vi "ME_acquire_12_DeltaForce_Daq.vi"() -> ()   [LabVIEW 2015]
doc: "Use this template to build a producer/consumer design pattern. Use this template when you need to execute a process, such as data analysis, when a data source, such as a triggered acquisition, produces data at an uneven rate and you need to execute the process when the data becomes available."
uses:
  Mode.ctl
  oxford_driver/Oxford Drivers/BUSGEN.LLB/OxfordAddress.ctl
  <vilib>/Analysis/baseanly.llb/Mean (DBL).vi
  <vilib>/DAQmx/read.llb/DAQmx Read (Analog 1D DBL 1Chan NSamp).vi
  <vilib>/Utility/file.llb/Write Delimited Spreadsheet (DBL).vi
  <vilib>/DAQmx/create/channels.llb/DAQmx Create Channel (AI-Voltage-Basic).vi
  <vilib>/DAQmx/configure/timing.llb/DAQmx Timing (Sample Clock).vi
  <vilib>/DAQmx/miscellaneous.llb/DAQmx Fill In Error Info.vi
  <vilib>/express/express arith-compare/Formula/XNode/ExpressFormulaBlockNode.xnode
  <vilib>/Analysis/NI_AALBase.lvlib
panel:
  out "mean":dbl format="%0.6f"
  out "remaining elements":T1(array[cluster])
  in  "Number of Samples":i32=100
  in  "Sample Rate":dbl=1000.0
  in  "Terminal Configuration":i32(ring)=-1 items=["default"=-1, "RSE"=10083, "NRSE"=10078, "Differential"=10106, "Pseudodifferential"=12529]
  in  "Max Voltage":dbl=5.0
  in  "Min Voltage":dbl=-5.0
  in  "Physical Channel":tag="Dev1/ai0"
  out "MagnetoRes (Ohm)":dbl
  in  "Averaged dt":dbl[][](array[numeric])
  in  "Averaged P(B)":dbl[][](array[numeric])
  out "LockInR":dbl
  out "deltaUaux":dbl
  out "Actual Voltage (V)":dbl caption="Actual AuxV" step=0.1
  in  "Stop":bool
  out "SaveSweep":bool=TRUE
  out "Measurement File_dn":path
  out "Measurement File_up":path
  out "Measurement File_average":path
  out "Actual Polarization":dbl
  in  "Reset IB?":bool
  in  "First?":bool
  in  "Save Period":dbl=1.0
  out "Averaged I(B)":dbl[][](array[numeric])
  out "P(uC/mm^2)":dbl[](array[numeric])
  in  "Sweep":bool
  out "Offset array":dbl[](array[numeric])
  in  "stop 2":bool
  in  "dB":dbl=0.005
  in  "Dwell Time (ms)":u32=1
  out "appended array":dbl[][](array[numeric])
  out "Actual B Field (T)":dbl
  out "Actual Temperature (K)":dbl
  out "Actual Current (pA)":dbl
  in  "Tab Control":T2(tab)
  in  "Max temperature (K)":dbl=20.0
  in  "Min Temperature (K)":dbl=4.5
  out "P(T)":cluster{"yi":dbl[], dbl[]}(graph)
  out "I(T)":cluster{dbl[], dbl[]}(graph)
  in  "Set temperature (K)":dbl=4.5
  in  "Temp Ramping Rate (K/min)":dbl=10.0
  in  "Heater Range":enum16{"Off", "Low", "Medium", "High"}(ring)
  in  "Heater On/Off":bool
  out "Setpoint Temperature (K)":dbl
  in  "FileName":string
  out "Step Temp":bool
  out "j":i32
  out "i":i32
  in  "Max Countl":i32
  in  "Record ALL":bool
  in  "Sweep Rate Array":dbl[](array[numeric])=[2.0, 1.0, 0.5, 0.1, 0.05, 9.0, 10.0, 11.0, 12.0]
  out "I(B) 3":cluster{dbl[], dbl[]}[](graph)
  in  "Go to Set":bool
  in  "Set Field (T)":dbl
  in  "Field To Zero":bool
  in  "Sweep Rate (T/min)":dbl=2.0 format="%.6f"
  in  "Min Field (T)":dbl
  in  "Max Field (T)":dbl=0.15
  out "Up/Down":bool
  out "I(B) /Averaged/":cluster{"B array":dbl[], dbl[]}[](graph)
  in  "Temperature Array":dbl[](array[numeric])=[4.5, 5.0, 6.0, 7.0, 8.0, 9.0, 10.0, 11.0, 12.0]
  out "New":bool=TRUE
  out "Step Rate":bool
  out "Finished":bool=TRUE
  in  "Directory":string
  out "Wait (s)":dbl
  in  "secs to wait":dbl=180.0
  in  "Max count array":i32[](array[numeric])=[2, 1, 0, 0, 0, 9, 10, 11, 12]
  out "Target Field":dbl
  out "P(B) /Averaged/":cluster{"B array":dbl[], dbl[]}[](graph)
  out "P(B)":cluster{"yi":dbl[], dbl[]}(graph)
  in  "Measure Noise":bool
  in  "Cycles":i32
  in  "maximum value":dbl=10.0 format="%0.2f"
  in  "minimum value":dbl=-10.0 format="%0.2f"
  in  "physical channels":tag="Dev1/ai1"
  out "PSD (pA/Hz^1/2) Peaks Removed":cluster{"f0":dbl, "df":dbl, "magnitude":dbl[]}(graph)
  out "PSD (pA/Hz^1/2)":cluster{"f0":dbl, "df":dbl, "magnitude":dbl[]}(graph)
  out "Current (pA) Filtered":waveform(dbl)(graph)
  out "Current (pA)":dbl[](graph)
  in  "Samples per channel":i32=1000
  in  "Rate":dbl=1000.0 format="%0.2f"
  in  "Cut-Off Frequency":dbl=100.0 caption="Lower Cut-Off"
  in  "Filter On":bool
  in  "Lock_in_Amplifier":refnum<visa-resource-name>="GPIB0::5::INSTR"
  out "Dc offset":dbl
  in  "Calibrate":bool
  in  "IV converter":refnum<visa-resource-name>="GPIB0::20::INSTR"
  in  "Magnetic Field":refnum<visa-resource-name>="GPIB0::21::INSTR"
  out "Time Lag":dbl=0.0500025749206543
  in  "Lake Shore":refnum<visa-resource-name>="GPIB0::11::INSTR"
  in  "Temp Refresh (s)":dbl=0.1
  in  "Sampling rate (Hz)":dbl=10.0
  in  "Gain (V/A)":dbl=1000000000.0
  in  "Sample area (mm^2)":dbl=3.9
  out "B_V":cluster{dbl[], "Best Linear Fit":dbl[]}[](graph)=[{[-0.00854253601, 0.00626134724, 0.0219834428, 0.0379117736, 0.0535871506, 0.0694316728, 0.0851615152, 0.100816481, 0.116478038, 0.132148461, 0.147876163, 0.16341701, 0.178976744, 0.194563632, 0.210251739, 0.225738944, 0.241298253, 0.256806034, 0.272344374, 0.287933477, 0.303494709, 0.318997125, 0.334591297, 0.350146681, 0.365618053, 0.380940961, 0.39666457, 0.412213675, 0.427724671, 0.443221444, 0.458760641, 0.474360042, 0.489915118, 0.505330598, 0.520967119, 0.536347531, 0.551813711, 0.567441155, 0.582995861, 0.598507522, 0.614041988, 0.629563151, 0.645106262, 0.660611914, 0.676136149, 0.691553948, 0.7071244, 0.72262999, 0.738171137, 0.753700392, 0.76919513, 0.784778028, 0.800215944, 0.8156961, 0.831325434, 0.846852183, 0.862326812, 0.877819169, 0.893312568, 0.90888536, 0.924354789], "Best Linear Fit"=[0.0, 0.005, 0.01, 0.015, 0.02, 0.025, 0.03, 0.035, 0.04, 0.045, 0.05, 0.055, 0.06, 0.065, 0.07, 0.075, 0.08, 0.085, 0.09, 0.095, 0.1, 0.105, 0.11, 0.115, 0.12, 0.125, 0.13, 0.135, 0.14, 0.145, 0.15, 0.155, 0.16, 0.165, 0.17, 0.175, 0.18, 0.185, 0.19, 0.195, 0.2, 0.205, 0.21, 0.215, 0.22, 0.225, 0.23, 0.235, 0.24, 0.245, 0.25, 0.255, 0.26, 0.265, 0.27, 0.275, 0.28, 0.285, 0.29, 0.295, 0.3]}, {[-0.00854253601, 0.00626134724, 0.0219834428, 0.0379117736, 0.0535871506, 0.0694316728, 0.0851615152, 0.100816481, 0.116478038, 0.132148461, 0.147876163, 0.16341701, 0.178976744, 0.194563632, 0.210251739, 0.225738944, 0.241298253, 0.256806034, 0.272344374, 0.287933477, 0.303494709, 0.318997125, 0.334591297, 0.350146681, 0.365618053, 0.380940961, 0.39666457, 0.412213675, 0.427724671, 0.443221444, 0.458760641, 0.474360042, 0.489915118, 0.505330598, 0.520967119, 0.536347531, 0.551813711, 0.567441155, 0.582995861, 0.598507522, 0.614041988, 0.629563151, 0.645106262, 0.660611914, 0.676136149, 0.691553948, 0.7071244, 0.72262999, 0.738171137, 0.753700392, 0.76919513, 0.784778028, 0.800215944, 0.8156961, 0.831325434, 0.846852183, 0.862326812, 0.877819169, 0.893312568, 0.90888536, 0.924354789], "Best Linear Fit"=[-0.00022554388023060128, 0.004536267537808887, 0.009593430775915074, 0.014716931562355689, 0.01975906732634002, 0.024855610270593523, 0.029915265354287977, 0.03495083565949541, 0.03998852608757118, 0.045029068349812316, 0.05008803495326229, 0.055086897848955874, 0.060091835929837946, 0.06510550835596321, 0.07015173884687344, 0.07513334727738563, 0.08013814865293042, 0.08512637555172443, 0.0901244320467579, 0.09513881694893507, 0.10014423687592358, 0.10513073807087174, 0.11014675346564809, 0.1151502923271957, 0.12012680792099008, 0.1250555686413888, 0.1301132186920259, 0.13511473785283767, 0.14010399888730068, 0.14508868495702945, 0.1500870171143548, 0.15510471446726903, 0.16010815425765457, 0.16506669165212906, 0.17009632901003072, 0.1750435864450521, 0.18001843198211442, 0.1850451496356715, 0.19004847041199868, 0.1950379453501071, 0.20003475573578386, 0.20502728708357412, 0.21002687821664084, 0.21501442030211, 0.220007939788244, 0.2249672231113706, 0.22997560874002893, 0.23496313088260184, 0.23996209027618054, 0.24495722449359253, 0.24994125598600042, 0.2549536449902534, 0.25991939913989753, 0.2648987401917687, 0.26992606578200207, 0.2749203939204135, 0.2798979571595809, 0.2848812227804405, 0.2898648235706211, 0.2948739618827834, 0.2998498524919418]}]
  out "V_I":cluster{dbl[], "Best Linear Fit":dbl[]}[](graph)=[{[0.0, 0.035, 0.069, 0.104, 0.138, 0.173, 0.208, 0.242, 0.277, 0.311, 0.346, 0.38, 0.415, 0.45, 0.484, 0.519, 0.553, 0.588, 0.623, 0.657, 0.692, 0.726, 0.761, 0.796, 0.83, 0.865, 0.899, 0.934, 0.969, 1.003, 1.038, 1.072, 1.107, 1.141, 1.176, 1.211, 1.245, 1.28, 1.314, 1.349, 1.384, 1.418, 1.453, 1.487, 1.522, 1.557, 1.591, 1.626, 1.66, 1.695, 1.73, 1.764, 1.799, 1.833, 1.868, 1.902, 1.937, 1.972, 2.006, 2.041, 2.075], "Best Linear Fit"=[-0.00854253601, 0.00626134724, 0.0219834428, 0.0379117736, 0.0535871506, 0.0694316728, 0.0851615152, 0.100816481, 0.116478038, 0.132148461, 0.147876163, 0.16341701, 0.178976744, 0.194563632, 0.210251739, 0.225738944, 0.241298253, 0.256806034, 0.272344374, 0.287933477, 0.303494709, 0.318997125, 0.334591297, 0.350146681, 0.365618053, 0.380940961, 0.39666457, 0.412213675, 0.427724671, 0.443221444, 0.458760641, 0.474360042, 0.489915118, 0.505330598, 0.520967119, 0.536347531, 0.551813711, 0.567441155, 0.582995861, 0.598507522, 0.614041988, 0.629563151, 0.645106262, 0.660611914, 0.676136149, 0.691553948, 0.7071244, 0.72262999, 0.738171137, 0.753700392, 0.76919513, 0.784778028, 0.800215944, 0.8156961, 0.831325434, 0.846852183, 0.862326812, 0.877819169, 0.893312568, 0.90888536, 0.924354789]}, {[0.0, 0.035, 0.069, 0.104, 0.138, 0.173, 0.208, 0.242, 0.277, 0.311, 0.346, 0.38, 0.415, 0.45, 0.484, 0.519, 0.553, 0.588, 0.623, 0.657, 0.692, 0.726, 0.761, 0.796, 0.83, 0.865, 0.899, 0.934, 0.969, 1.003, 1.038, 1.072, 1.107, 1.141, 1.176, 1.211, 1.245, 1.28, 1.314, 1.349, 1.384, 1.418, 1.453, 1.487, 1.522, 1.557, 1.591, 1.626, 1.66, 1.695, 1.73, 1.764, 1.799, 1.833, 1.868, 1.902, 1.937, 1.972, 2.006, 2.041, 2.075], "Best Linear Fit"=[-0.007846580254753975, 0.007882153481927697, 0.02316149482613275, 0.03889022856281441, 0.054169569907019474, 0.06989830364370113, 0.08562703738038281, 0.10090637872458785, 0.11663511246126955, 0.1319144538054746, 0.14764318754215625, 0.1629225288863613, 0.17865126262304296, 0.19437999635972467, 0.2096593377039297, 0.22538807144061138, 0.24066741278481643, 0.25639614652149806, 0.27212488025817977, 0.2874042216023848, 0.3031329553390665, 0.31841229668327153, 0.3341410304199532, 0.3498697641566349, 0.3651491055008399, 0.3808778392375216, 0.39615718058172666, 0.4118859143184083, 0.42761464805509, 0.442893989399295, 0.45862272313597674, 0.4739020644801818, 0.48963079821686345, 0.5049101395610684, 0.5206388732977502, 0.5363676070344319, 0.5516469483786369, 0.5673756821153185, 0.5826550234595236, 0.5983837571962053, 0.6141124909328869, 0.629391832277092, 0.6451205660137737, 0.6603999073579787, 0.6761286410946604, 0.691857374831342, 0.7071367161755471, 0.7228654499122288, 0.7381447912564338, 0.7538735249931156, 0.7696022587297972, 0.7848816000740022, 0.8006103338106839, 0.815889675154889, 0.8316184088915707, 0.8468977502357756, 0.8626264839724573, 0.878355217709139, 0.893634559053344, 0.9093632927900257, 0.9246426341342309]}]
  out "B0 (T)":dbl=0.0025222449819540214
  out "B/V (T/V)":dbl=0.321659617116981
  out "I0 (A)":dbl=-0.007846580254753975
  out "V/I (Ohm)":dbl=0.44939239247661916
  in  "Offset?":bool
  in  "Magnet":bool
  in  "Ramp":bool=TRUE
  out "MagnetoResistance (Ohm)":cluster{dbl[], dbl[]}(graph)
  in  "Temp/Magnetic Field":bool
  out "index":i8
  out "Read?":bool
  out "Magnetic Field (T)":dbl[](array[numeric])
  out "Reset":bool
  out "Measured Current (pA)":dbl[](array[numeric])
  out "Elapsed Time (s)":dbl[](array[numeric])
  out "Start time":timestamp
  in  "Enum":T3=enum."Process"
  out "B array":dbl[](array[numeric])
  in  "dB (T)":dbl=0.0025
  in  "Counter":i8
  out "L magnet (H)":dbl
  out "R magnet (mOhm)":dbl
  out "Actual Current (R0)":dbl
  out "Actual Field (T)":dbl
  out "Temperature array":dbl[](array[numeric])
  in  "New Measurement File":bool
  out "Measurement File":path
  out "refnum out":refnum<file>
  in  "Measuring":bool
  in  "Measure /Pause":bool
  in  "stop":bool
  # "DeltaForce"
  # "Discrete"
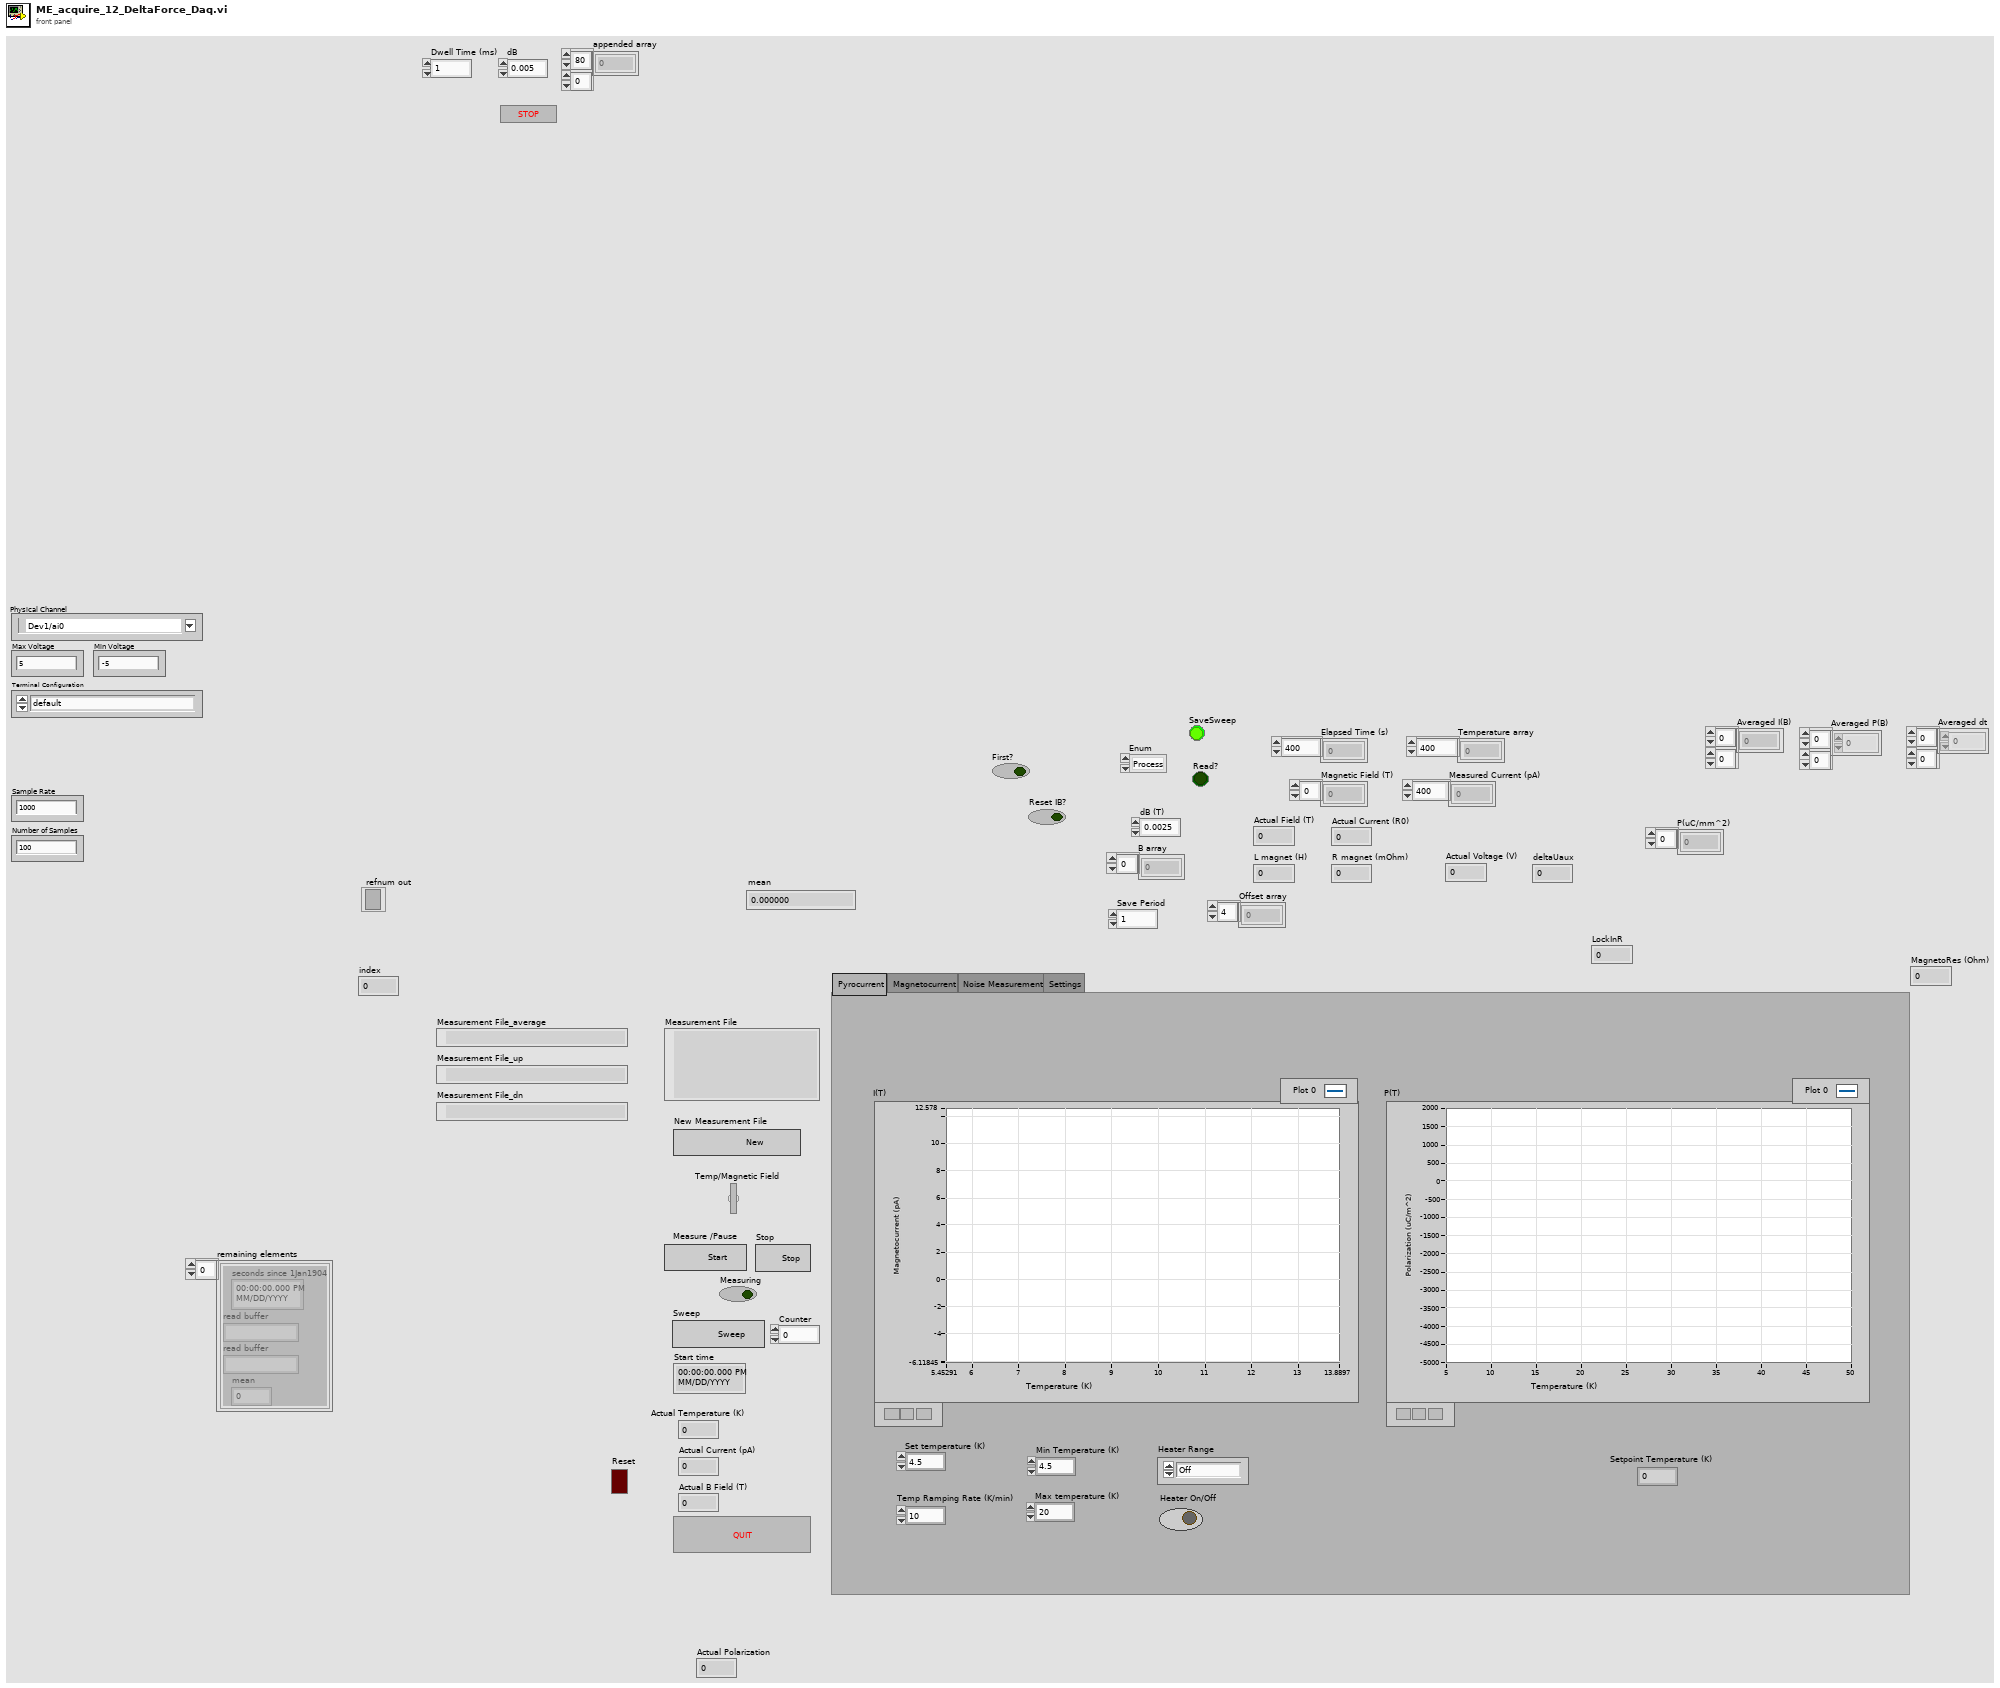
[diagram p1: front panel]
types:
  T1 = cluster{"seconds since 1Jan1904":timestamp, "read buffer":string, "read buffer":string, "mean":dbl}[]
  T2 = enum32{"Pyrocurrent", "Magnetocurrent", "Noise Measurement", "Settings"}
  T3 = typedef "Mode.ctl" = enum16{"Offset", "Process", "Sweep", "StepField", "Plot", "Save", "New", "Return", ""}
  T4 = cluster{"seconds since 1Jan1904":timestamp, "read buffer":string, "read buffer":string, "mean":dbl}
  T5 = enum16{"open", "replace", "create", "open or create", "replace or create", "replace or create with confirmation"}
  T6 = typedef "OxfordAddress.ctl" = cluster{"Com Port":i32, "ISOBUS Address":i32, "GPIB Address":i16, "Communication":enum16{"RS232", "ISOBUS", "GPIB", "Gateway"}}
  T7 = cluster{"B array":dbl[], "Averaged P(B) Out":dbl[]}
  T8 = cluster{"B array":dbl[], "Averaged I(B) out":dbl[]}
  T9 = cluster{"B array":dbl[], "Averaged P(B) Out":dbl[]}[]
  T10 = cluster{"B array":dbl[], "Averaged I(B) out":dbl[]}[]
  T11 = cluster{"I array out (A)":dbl[], "V array out (V)":dbl[]}
  T12 = cluster{"I array out (A)":dbl[], "Best Linear Fit":dbl[]}
  T13 = cluster{"V array out (V)":dbl[], "B array Out":dbl[]}
  T14 = cluster{"V array out (V)":dbl[], "Best Linear Fit 2":dbl[]}
  T15 = cluster{"I array out (A)":dbl[], "Best Linear Fit":dbl[]}[]
  T16 = cluster{"V array out (V)":dbl[], "Best Linear Fit 2":dbl[]}[]
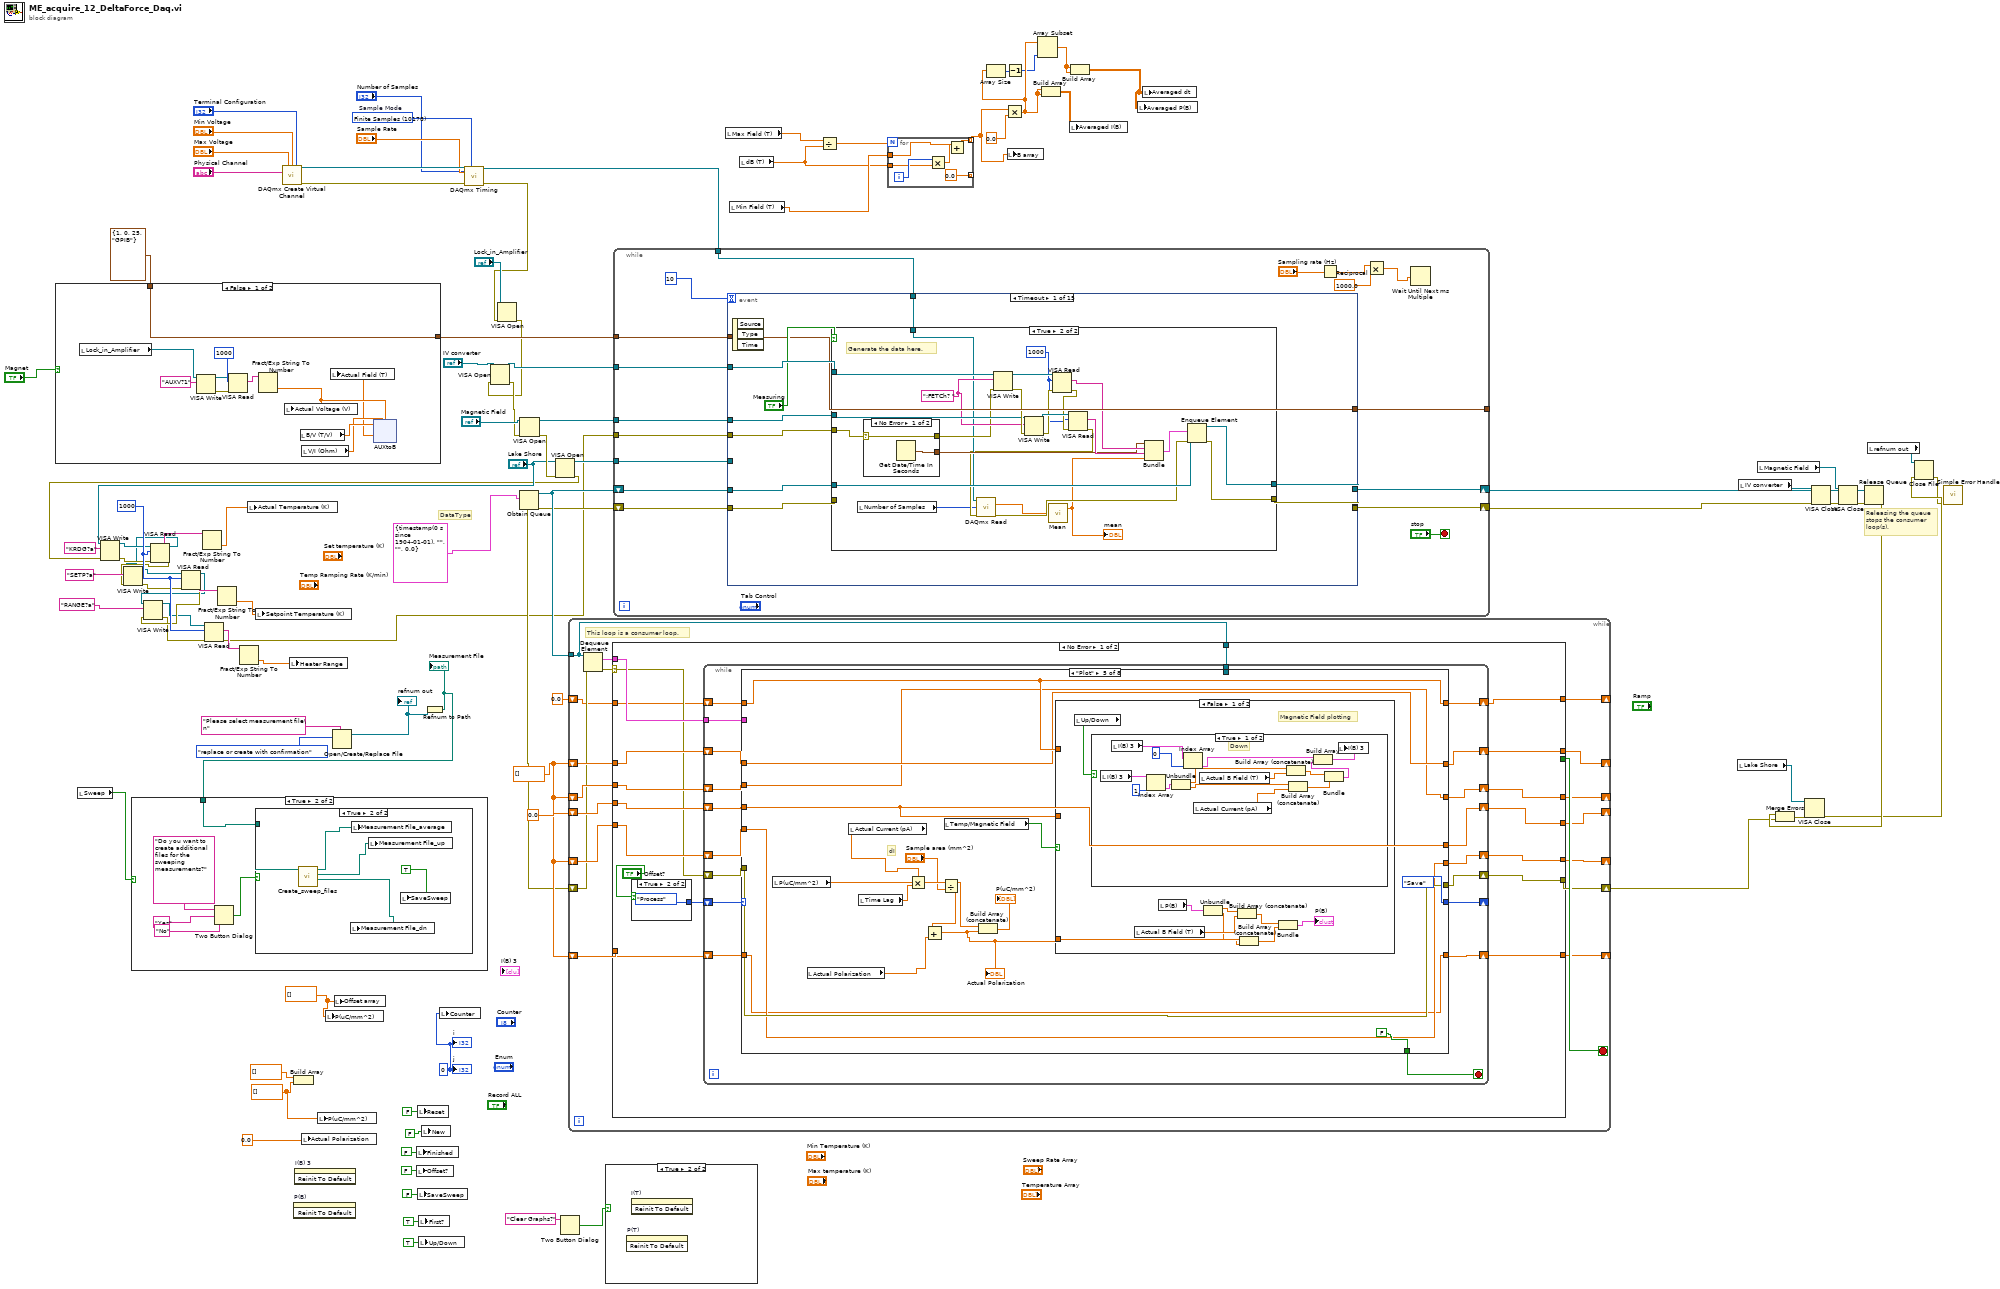
[diagram p0: block diagram]
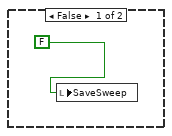
[diagram p4: hidden frame]
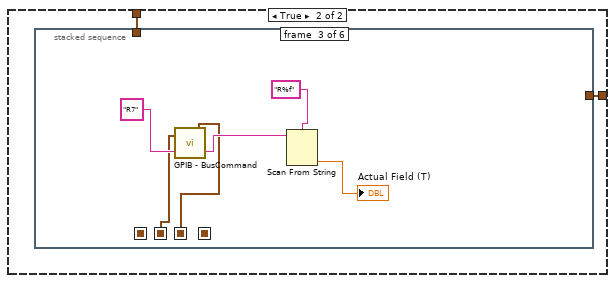
[diagram p5: hidden frame]
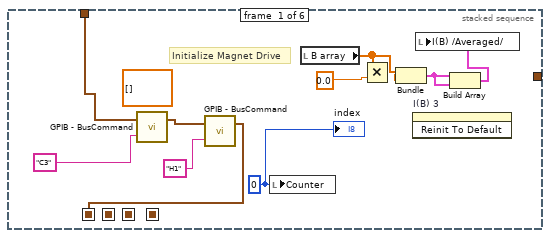
[diagram p6: hidden frame]
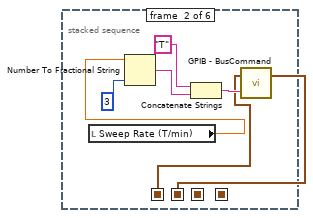
[diagram p7: hidden frame]
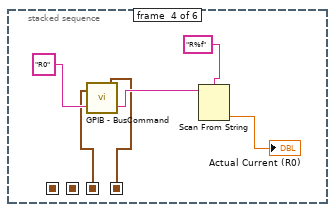
[diagram p8: hidden frame]
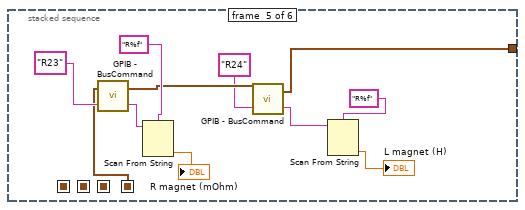
[diagram p9: hidden frame]
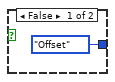
[diagram p11: hidden frame]
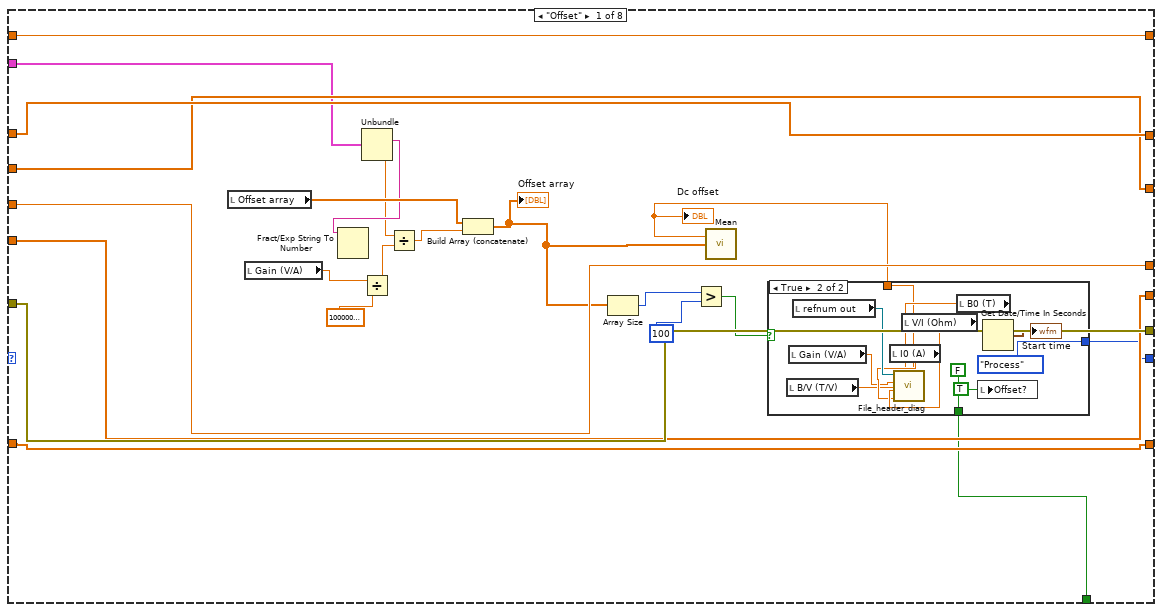
[diagram p12: hidden frame]
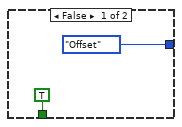
[diagram p13: hidden frame]
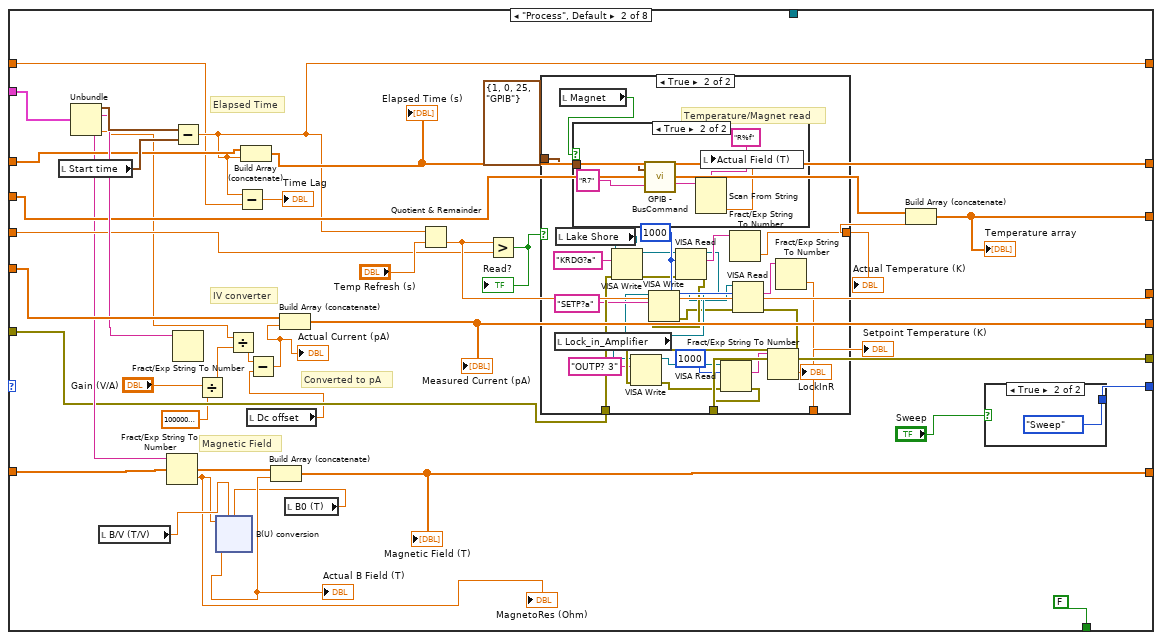
[diagram p14: hidden frame]
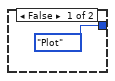
[diagram p15: hidden frame]
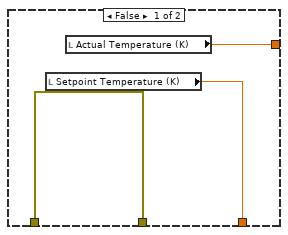
[diagram p16: hidden frame]
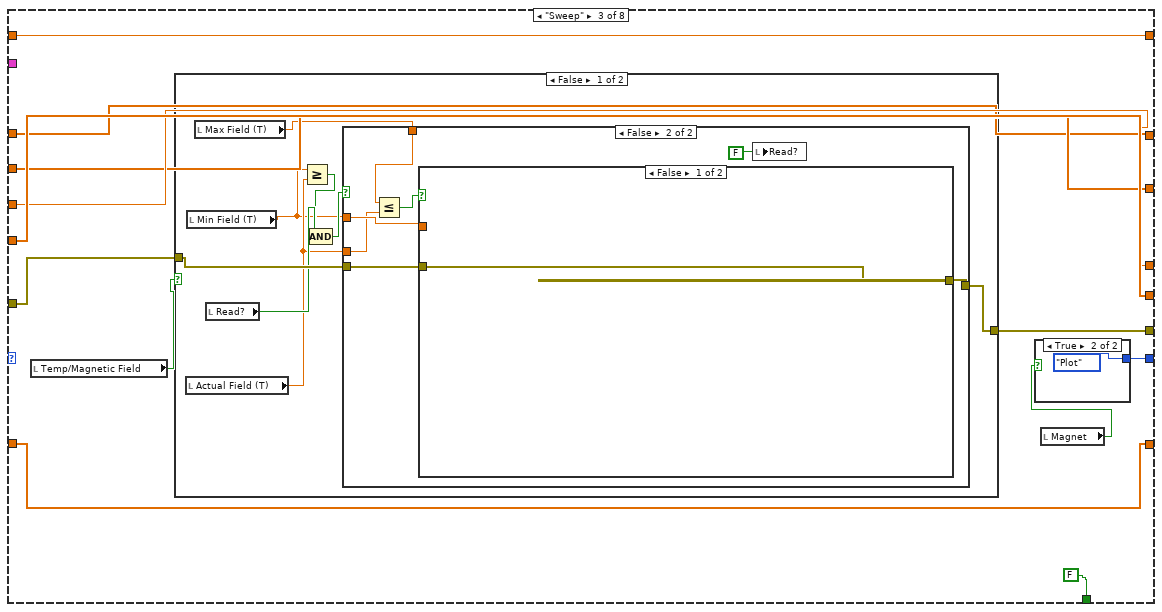
[diagram p18: hidden frame]
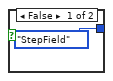
[diagram p19: hidden frame]
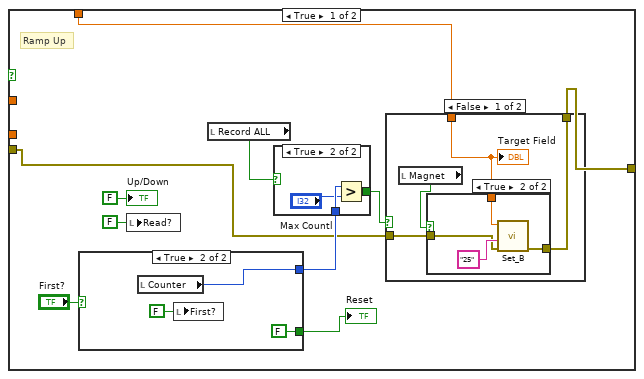
[diagram p20: hidden frame]
diagram:
  w9 = 10178 items=["Finite Samples"=10178, "Continuous Samples"=10123, "Hardware Timed Single Point"=12522]  # Sample Mode
  w39 = u32 1000 ("byte count")
  w50 = 0 ("j")
  w47 = dbl[] []
  w65 = dbl[] []
  w71 = dbl[] []
  # "DataType"
  # "Releasing the queue stops the consumer loop(s)."
  n1 = case shown="False" "Magnet" {
    tunnel: T6 {"Com Port"=1, "ISOBUS Address"=0, "GPIB Address"=25, "Communication"=enum."GPIB"} ("Address") -> [w107 w121]
    tunnel: [w107 w120] -> w77
    frame False {
      n2 = local read "Lock_in_Amplifier"() -> (w101:refnum<visa-resource-name>)
      n3 = VISA Write(VISA resource name=w101, write buffer="AUXV?1") -> (VISA resource name out=w102:refnum<visa-resource-name>, error out=w106:errorcluster)  [unwired: 1 in, 1 out]
      n4 = VISA Read(VISA resource name=w102, byte count=u32 1000, error in (no error)=w106) -> (read buffer=w105:string)  [unwired: 3 out]
      n5 = Fract/Exp String To Number(string=w105) -> (number=w98:dbl)  [unwired: 3 in, 1 out]
      n6 = local write "Actual Voltage (V)"(w98) -> ()
      n7 = local read "B/V (T/V)"() -> (w100:dbl)
      n8 = local read "V/I (Ohm)"() -> (w99:dbl)
      n9 = xnode "AUXtoB"("BpV"=w100, "Rm"=w99, "Aux"=w98) -> ("Result"=w97:dbl)  [unwired: 1 in, 1 out]
      n10 = local write "Actual Field (T)"(w97) -> ()
    }
    frame True {
      n11 = stacked-sequence {
        seq-local: [w129 _ _ _ _ _] -> [_ w134 _ _ _ _]
        seq-local: [_ w133 _ _ _ _] -> [_ _ w141 _ _ _]
        seq-local: [_ _ w140 _ _ _] -> [_ _ _ w147 _ _]
        seq-local: [_ _ _ w146 _ _] -> [_ _ _ _ w158 _]
        tunnel: w121 -> [w131 _ _ _ _ _]
        tunnel: [_ _ _ _ w156 _] -> w120
        frame #0 {
          (unwired) dbl[][] []
          w127 = i8 0 ("Counter")
          # "Initialize Magnet Drive"
          n12 = call "GPIB - BusCommand.vi"("Command"="C3", "Address"=w131) -> ("Address(thru)"=w130:T6)  [unwired: 1 out]
          n13 = call "GPIB - BusCommand.vi"("Command"="H1", "Address"=w130) -> ("Address(thru)"=w129:T6)  [unwired: 1 out]
          n14 = local write "Counter"(w127) -> ()
          n15 = local read "B array"() -> (w125:dbl[])
          n16 = Multiply(x=w125, y=0.0) -> (x*y=w124:dbl[])
          n17 = Bundle("B array"=w125, w124) -> (w123:cluster{"B array":dbl[], dbl[]})  [unwired: 1 in]
          n18 = invoke on="I(B) 3" class="XYGraph (strict)" method="Reinit To Default"() -> ()  [unwired: 3 in, 3 out]
          n19 = Build Array(w123, w123) -> (w122:cluster{"B array":dbl[], dbl[]}[])
          n20 = local write "I(B) /Averaged/"(w122) -> ()
          "index" <- w127
        }
        frame #1 {
          n21 = local read "Sweep Rate (T/min)"() -> (w135:dbl)
          n22 = Number To Fractional String(number=w135, precision (6)=i16 3) -> (F-format string=w137:string)  [unwired: 2 in]
          n23 = Concatenate Strings("T" ("format string"), w137) -> (w136:string)
          n24 = call "GPIB - BusCommand.vi"("Command"=w136, "Address"=w134) -> ("Address(thru)"=w133:T6)  [unwired: 1 out]
        }
        frame #2 {
          n25 = call "GPIB - BusCommand.vi"("Command"="R7" ("format string"), "Address"=w141) -> ("Reply"=w145:string, "Address(thru)"=w140:T6)
          n26 = Scan From String(format string="R%f" ("remaining string"), input string=w145) -> (output 1=→"Actual Field (T)":dbl)  [unwired: 3 in, 3 out]
        }
        frame #3 {
          n27 = call "GPIB - BusCommand.vi"("Command"="R0" ("format string"), "Address"=w147) -> ("Reply"=w151:string, "Address(thru)"=w146:T6)
          n28 = Scan From String(format string="R%f" ("remaining string"), input string=w151) -> (output 1=→"Actual Current (R0)":dbl)  [unwired: 3 in, 3 out]
        }
        frame #4 {
          n29 = call "GPIB - BusCommand.vi"("Command"="R23" ("format string"), "Address"=w158) -> ("Reply"=w162:string, "Address(thru)"=w157:T6)
          n30 = Scan From String(format string="R%f" ("remaining string"), input string=w162) -> (output 1=→"R magnet (mOhm)":dbl)  [unwired: 3 in, 3 out]
          n31 = call "GPIB - BusCommand.vi"("Command"="R24" ("format string"), "Address"=w157) -> ("Reply"=w154:string, "Address(thru)"=w156:T6)
          n32 = Scan From String(format string="R%f" ("remaining string"), input string=w154) -> (output 1=→"L magnet (H)":dbl)  [unwired: 3 in, 3 out]
        }
        frame #5 {
        }
      }
    }
  }
  n33 = local read "Sweep"() -> (w55:bool)
  n34 = call-poly <vilib>:"DAQmx Create Virtual Channel.vi"("maximum value"="Max Voltage", "minimum value"="Min Voltage", "input terminal configuration"="Terminal Configuration", "physical channels"="Physical Channel") -> ("task out"=w7:refnum<k21>, "error out"=w8:errorcluster)  [unwired: 10 in]
  n35 = Build Array(dbl[] [], w47) -> ()  [unwired: 1 out]
  n36 = invoke on="P(B)" class="XYGraph (strict)" method="Reinit To Default"() -> ()  [unwired: 3 in, 3 out]
  n37 = invoke on="I(B) 3" class="XYGraph (strict)" method="Reinit To Default"() -> ()  [unwired: 3 in, 3 out]
  n38 = local write "Actual Polarization"(0.0 ("Actual Polarization")) -> ()
  n39 = local write "P(uC/mm^2)"(w47) -> ()
  n40 = local write "P(uC/mm^2)"(w65) -> ()
  n41 = Open/Create/Replace File(prompt="Please select measurement file\n", operation (0:open)=T5."replace or create with confirmation") -> (refnum out=w74:refnum<file>)  [unwired: 4 in, 2 out]
  "refnum out" <- w74
  n42 = local write "Offset array"(w65) -> ()
  n43 = local write "Finished"(FALSE ("Finished")) -> ()
  n44 = local write "Offset?"(FALSE ("Offset?")) -> ()
  n45 = local write "Reset"(FALSE ("Reset")) -> ()
  n46 = local write "SaveSweep"(FALSE ("SaveSweep")) -> ()
  n47 = local write "First?"(TRUE ("First?")) -> ()
  n48 = local write "Up/Down"(TRUE ("Up/Down")) -> ()
  n49 = local write "New"(FALSE ("New")) -> ()
  n50 = Refnum to Path(1:w74) -> (0:w54:path)
  "Measurement File" <- w54
  n51 = case shown="True" w55 {
    tunnel: w54 -> [_ w163]
    frame False {
    }
    frame True {
      n52 = Two Button Dialog(message="Do you want to create additional files for the sweeping measurements?" ("string"), 1:"No" ("F button name (\"Cancel\")"), 2:"Yes" ("T button name (\"OK\")")) -> (T button?=w165:bool)
      n53 = case shown="True" w165 {
        tunnel: w163 -> [_ w173]
        frame False {
          n54 = local write "SaveSweep"(FALSE ("SaveSweep")) -> ()
        }
        frame True {
          n55 = call "Create_sweep_files.vi"("Measurement File"=w173) -> ("Path 3"=w170:path, "Path 2"=w171:path, "Path"=w172:path)  [unwired: 8 in]
          n56 = local write "Measurement File_dn"(w170) -> ()
          n57 = local write "Measurement File_average"(w172) -> ()
          n58 = local write "Measurement File_up"(w171) -> ()
          n59 = local write "SaveSweep"(TRUE) -> ()
        }
      }
    }
  }
  n60 = local write "Counter"(w50) -> ()
  n61 = call-poly <vilib>:"DAQmx Timing.vi"("task/channels in"=w7, "sample mode"=w9, "samples per channel"="Number of Samples", "rate"="Sample Rate", "error in"=w8) -> ("task out"=w11:refnum<k21>, "error out"=w12:errorcluster)  [unwired: 9 in]
  n62 = VISA Open(error in (no error)=w12, VISA resource name="Lock_in_Amplifier") -> (error out=w22:errorcluster)  [unwired: 3 in, 1 out]
  n63 = VISA Open(error in (no error)=w22, VISA resource name="IV converter") -> (VISA resource name=w91:refnum<visa-resource-name>, error out=w93:errorcluster)  [unwired: 3 in]
  n64 = Obtain Queue(element data type=T4 {"seconds since 1Jan1904"=timestamp(0 s since 1904-01-01), "read buffer"="", "read buffer"="", "mean"=0.0} ("output cluster")) -> (queue out=w96:refnum<queue>, error out=w69:errorcluster)  [unwired: 4 in, 1 out]
  n65 = VISA Open(error in (no error)=w93, VISA resource name="Magnetic Field") -> (VISA resource name=w90:refnum<visa-resource-name>, error out=w72:errorcluster)  [unwired: 3 in]
  n66 = VISA Open(error in (no error)=w72, VISA resource name="Lake Shore") -> (VISA resource name=w67:refnum<visa-resource-name>, error out=w36:errorcluster)  [unwired: 3 in]
  n67 = VISA Write(VISA resource name="Lake Shore", write buffer="KRDG?a", error in (no error)=w36) -> (VISA resource name out=w33:refnum<visa-resource-name>, error out=w32:errorcluster)  [unwired: 1 out]
  n68 = VISA Read(VISA resource name=w33, byte count=w39, error in (no error)=w32) -> (VISA resource name out=w30:refnum<visa-resource-name>, read buffer=w44:string, error out=w31:errorcluster)  [unwired: 1 out]
  n69 = VISA Write(VISA resource name=w30, write buffer="SETP?a", error in (no error)=w31) -> (VISA resource name out=w29:refnum<visa-resource-name>, error out=w28:errorcluster)  [unwired: 1 out]
  n70 = VISA Read(VISA resource name=w29, byte count=w39, error in (no error)=w28) -> (VISA resource name out=w26:refnum<visa-resource-name>, read buffer=w43:string, error out=w27:errorcluster)  [unwired: 1 out]
  n71 = VISA Write(VISA resource name=w26, write buffer="RANGE?a", error in (no error)=w27) -> (VISA resource name out=w24:refnum<visa-resource-name>, error out=w25:errorcluster)  [unwired: 1 out]
  n72 = Fract/Exp String To Number(string=w44) -> (number=w42:dbl)  [unwired: 3 in, 1 out]
  n73 = VISA Read(VISA resource name=w24, byte count=w39, error in (no error)=w25) -> (read buffer=w38:string, error out=w35:errorcluster)  [unwired: 2 out]
  n74 = Fract/Exp String To Number(string=w43) -> (number=w41:dbl)  [unwired: 3 in, 1 out]
  n75 = Fract/Exp String To Number(string=w38) -> (number=w34:dbl)  [unwired: 3 in, 1 out]
  n76 = local write "Actual Temperature (K)"(w42) -> ()
  n77 = local write "Setpoint Temperature (K)"(w41) -> ()
  n78 = local write "Heater Range"(w34) -> ()
  n79 = Two Button Dialog(message="Clear Graphs?") -> (T button?=w49:bool)  [unwired: 2 in]
  n80 = while {
    tunnel: w96 -> [w174]
    shift-right: [w187] -> _
    shift-left: w71 -> [w186]
    shift-right: [w185] -> _
    shift-left: w71 -> [w184]
    shift-right: [w183] -> _
    shift-left: w71 -> [w182]
    shift-right: [w181] -> _
    shift-left: 0.0 -> [w180]
    shift-right: [w179] -> _
    shift-left: w71 -> [w178]
    shift-right: [w188] -> w82
    shift-left: w69 -> [w177]
    shift-right: [w176] -> _
    shift-left: 0.0 -> [w175]
    stop <- w189 stop-if-true
    # "This loop is a consumer loop."
    n81 = Dequeue Element(queue=w174, error in (no error)=w177) -> (element=w190:T4, error out=w191:errorcluster)  [unwired: 1 in, 2 out]
    n82 = case shown="No Error" w191 {
      selector: w191 -> [w197 w860]
      tunnel: w190 -> [w208 _]
      tunnel: [_ TRUE] -> w189
      tunnel: [w196 w860] -> w188
      tunnel: [w207 w859] -> w187
      tunnel: w186 -> [w206 w859]
      tunnel: [w205 w856] -> w185
      tunnel: w184 -> [w204 w856]
      tunnel: [w203 w855] -> w183
      tunnel: w182 -> [w202 w855]
      tunnel: [w201 w857] -> w181
      tunnel: w180 -> [w200 w857]
      tunnel: [w199 w858] -> w179
      tunnel: w178 -> [w198 w858]
      tunnel: [w195 w854] -> w176
      tunnel: w175 -> [w194 w854]
      tunnel: w174 -> [w192 _]
      frame No Error {
        n83 = case shown="True" "Offset?" {
          tunnel: [Mode."Offset" ("Enum") Mode."Process" ("Enum")] -> w209
          frame False {
          }
          frame True {
          }
        }
        n84 = while {
          shift-right: [w218] -> _
          shift-left: w209 -> [w230]
          tunnel: w208 -> [w229]
          shift-right: [w228] -> w207
          shift-left: w206 -> [w227]
          shift-right: [w220] -> w199
          shift-left: w198 -> [w219]
          shift-right: [w222] -> w201
          shift-left: w200 -> [w221]
          shift-right: [w226] -> w205
          shift-left: w204 -> [w225]
          shift-right: [w216] -> w196
          shift-left: w197 -> [w217]
          shift-right: [w224] -> w203
          shift-left: w202 -> [w223]
          shift-right: [w214] -> w195
          shift-left: w194 -> [w213]
          tunnel: w192 -> [w212]
          stop <- w215 stop-if-true
          n85 = case shown="\"Plot\"" w230 {
            selector: w230 -> [_ _ _ _ _ _ _ w847]
            tunnel: w229 -> [w246 w302 _ _ _ _ _ _]
            tunnel: [w252 w299 w357 w472 w534 w615 w696 w852] -> w228
            tunnel: w227 -> [w252 w292 w357 w472 w534 w611 w696 w852]
            tunnel: [w247 w298 w360 w469 w536 w617 w694 w849] -> w226
            tunnel: w225 -> [w247 w297 w360 w469 w536 w612 w694 w849]
            tunnel: [w248 w295 w362 w467 w531 w618 w692 w846] -> w224
            tunnel: w223 -> [w248 w294 w362 w467 w531 w613 w692 w846]
            tunnel: [w250 w291 w359 w470 w532 w621 0.0 w850] -> w222
            tunnel: w221 -> [w250 w290 w359 w470 w532 w621 _ w850]
            tunnel: [w251 w287 w358 w471 w533 w616 w695 w851] -> w220
            tunnel: w219 -> [w251 w288 w358 w471 w533 w614 w695 w851]
            tunnel: [w236 w285 w355 Mode."Plot" ("Enum") Mode."Save" ("Enum") w622 Mode."Return" ("Enum") w847] -> w218
            tunnel: w217 -> [w249 w283 w364 w464 w539 w620 w688 w848]
            tunnel: [w249 w282 w363 w463 w539 w620 w687 w848] -> w216
            tunnel: [w232 FALSE FALSE FALSE FALSE w609 TRUE TRUE] -> w215
            tunnel: [w235 w279 w356 w465 w535 w619 0.0 w853] -> w214
            tunnel: w213 -> [w235 w278 w356 w465 w535 w619 _ w853]
            tunnel: w212 -> [_ _ _ _ _ _ w686 _]
            frame "Offset" {
              n86 = local read "Offset array"() -> (w241:dbl[])
              n87 = local read "Gain (V/A)"() -> (w245:dbl)
              n88 = Unbundle(w246) -> ("read buffer"=w234:string, "mean"=w231:dbl)  [unwired: 2 out]
              n89 = Fract/Exp String To Number(string=w234) -> ()  [unwired: 3 in, 2 out]
              n90 = Divide(x=w245, y=1000000000000.0) -> (x/y=w243:dbl)
              n91 = Divide(x=w231, y=w243) -> (x/y=w242:dbl)
              n92 = Build Array (concatenate)(w241, w242) -> (w237:dbl[])
              "Offset array" <- w237
              n93 = Array Size(array=w237) -> (size(s)=w240:i32)
              n94 = Greater?(x=w240, y=100) -> (0:w238:bool)
              n95 = call-poly <vilib>:"Mean.vi"("X"=w237) -> ("mean"=w233:dbl)  [unwired: 1 out]
              "Dc offset" <- w233
              n96 = case shown="True" w238 {
                tunnel: [Mode."Offset" ("Enum") Mode."Process" ("Enum")] -> w236
                tunnel: w233 -> [_ w257]
                tunnel: [TRUE FALSE] -> w232
                frame False {
                }
                frame True {
                  n97 = local read "B/V (T/V)"() -> (w258:dbl)
                  n98 = local read "Gain (V/A)"() -> (w259:dbl)
                  n99 = local read "refnum out"() -> (w263:refnum<file>)
                  n100 = local read "I0 (A)"() -> (w261:dbl)
                  n101 = local read "V/I (Ohm)"() -> (w262:dbl)
                  n102 = local read "B0 (T)"() -> (w260:dbl)
                  n103 = call "File_header_diag.vi"("OFFSET"=w257, "B0"=w260, "B/V"=w258, "I0"=w261, "V/I"=w262, "Gain"=w259, "Byte Stream File in"=w263) -> ()  [unwired: 5 in]
                  n104 = local write "Offset?"(TRUE ("Offset?")) -> ()
                  n105 = Get Date/Time In Seconds() -> (seconds since 1Jan1904=→"Start time":timestamp)
                }
              }
            }
            frame "Process", Default {
              # "Converted to pA"
              # "Magnetic Field"
              # "IV converter"
              # "Elapsed Time"
              n106 = local read "Start time"() -> (w300:timestamp)
              n107 = Unbundle(w302) -> ("seconds since 1Jan1904"=w301:timestamp, "read buffer"=w296:string, "read buffer"=w284:string, "mean"=w266:dbl)
              n108 = local read "B/V (T/V)"() -> (w274:dbl)
              n109 = Fract/Exp String To Number(string=w284) -> (number=w267:dbl)  [unwired: 3 in, 1 out]
              "MagnetoRes (Ohm)" <- w267
              n110 = Subtract(x=w301, y=w300) -> (x-y=w279:dbl)
              n111 = Fract/Exp String To Number(string=w296) -> ()  [unwired: 3 in, 2 out]
              n112 = Divide(x="Gain (V/A)", y=1000000000000.0) -> (x/y=w277:dbl)
              n113 = Divide(x=w266, y=w277) -> (x/y=w272:dbl)
              n114 = Subtract(x=w279, y=w278) -> (x-y=→"Time Lag":dbl)
              n115 = Build Array (concatenate)(w292, w279) -> (w299:dbl[])
              "Elapsed Time (s)" <- w299
              n116 = local read "Dc offset"() -> (w270:dbl)
              n117 = Subtract(x=w272, y=w270) -> (x-y=w271:dbl)
              "Actual Current (pA)" <- w271
              n118 = Build Array (concatenate)(w297, w271) -> (w298:dbl[])
              "Measured Current (pA)" <- w298
              n119 = local read "B0 (T)"() -> (w273:dbl)
              n120 = xnode "B(U) conversion"("V"=w267, "BpV"=w274, "B0"=w273) -> ("Result"=w293:dbl)  [unwired: 1 in, 1 out]
              "Actual B Field (T)" <- w293
              n121 = Build Array (concatenate)(w294, w293) -> (w295:dbl[])
              "Magnetic Field (T)" <- w295
              n122 = Quotient & Remainder(x=w279, y="Temp Refresh (s)") -> (floor(x/y)=w291:dbl)  [unwired: 1 out]
              n123 = Greater?(x=w291, y=w290) -> (0:w289:bool)
              "Read?" <- w289
              n124 = case shown="True" w289 {
                tunnel: [w308 w333] -> w286
                tunnel: w283 -> [w309 w332]
                tunnel: [w309 w312] -> w282
                tunnel: T6 {"Com Port"=1, "ISOBUS Address"=0, "GPIB Address"=25, "Communication"=enum."GPIB"} ("Address") -> [_ w331]
                tunnel: [w307 w327] -> w268
                frame False {
                  n125 = local read "Setpoint Temperature (K)"() -> (w307:dbl)
                  n126 = local read "Actual Temperature (K)"() -> (w308:dbl)
                }
                frame True {
                  w328 = u32 1000 ("byte count")
                  # "Temperature/Magnet read"
                  n127 = local read "Lock_in_Amplifier"() -> (w316:refnum<visa-resource-name>)
                  n128 = local read "Lake Shore"() -> (w330:refnum<visa-resource-name>)
                  n129 = local read "Magnet"() -> (w319:bool)
                  n130 = case shown="True" w319 {
                    tunnel: w331 -> [_ w337]
                    frame False {
                    }
                    frame True {
                      n131 = call "GPIB - BusCommand.vi"("Command"="R7" ("format string"), "Address"=w337) -> ("Reply"=w338:string)  [unwired: 1 out]
                      n132 = Scan From String(format string="R%f" ("remaining string"), input string=w338) -> (output 1=w336:dbl)  [unwired: 3 in, 3 out]
                      n133 = local write "Actual Field (T)"(w336) -> ()
                    }
                  }
                  n134 = VISA Write(VISA resource name=w330, write buffer="KRDG?a", error in (no error)=w332) -> (VISA resource name out=w326:refnum<visa-resource-name>, error out=w324:errorcluster)  [unwired: 1 out]
                  n135 = VISA Read(VISA resource name=w326, byte count=w328, error in (no error)=w324) -> (VISA resource name out=w325:refnum<visa-resource-name>, read buffer=w334:string, error out=w323:errorcluster)  [unwired: 1 out]
                  n136 = VISA Write(VISA resource name=w325, write buffer="SETP?a", error in (no error)=w323) -> (VISA resource name out=w321:refnum<visa-resource-name>, error out=w322:errorcluster)  [unwired: 1 out]
                  n137 = Fract/Exp String To Number(string=w334) -> (number=w333:dbl)  [unwired: 3 in, 1 out]
                  n138 = VISA Read(VISA resource name=w321, byte count=w328, error in (no error)=w322) -> (read buffer=w320:string, error out=w318:errorcluster)  [unwired: 2 out]
                  n139 = VISA Write(VISA resource name=w316, write buffer="OUTP? 3", error in (no error)=w318) -> (VISA resource name out=w315:refnum<visa-resource-name>, error out=w317:errorcluster)  [unwired: 1 out]
                  n140 = VISA Read(VISA resource name=w315, byte count=u32 1000, error in (no error)=w317) -> (read buffer=w311:string, error out=w312:errorcluster)  [unwired: 2 out]
                  n141 = Fract/Exp String To Number(string=w311) -> (number=→"LockInR":dbl)  [unwired: 3 in, 1 out]
                  n142 = Fract/Exp String To Number(string=w320) -> (number=w327:dbl)  [unwired: 3 in, 1 out]
                }
              }
              "Actual Temperature (K)" <- w286
              "Setpoint Temperature (K)" <- w268
              n143 = Build Array (concatenate)(w288, w286) -> (w287:dbl[])
              "Temperature array" <- w287
              n144 = case shown="True" "Sweep" {
                tunnel: [Mode."Plot" ("Enum") Mode."Sweep" ("Enum")] -> w285
                frame False {
                }
                frame True {
                }
              }
            }
            frame "Sweep" {
              n145 = local read "Temp/Magnetic Field"() -> (w354:bool)
              n146 = case shown="False" w354 {
                tunnel: w364 -> [w373 w430]
                tunnel: [w372 w429] -> w363
                frame False {
                  n147 = local read "Actual Field (T)"() -> (w368:dbl)
                  n148 = local read "Min Field (T)"() -> (w367:dbl)
                  n149 = local read "Max Field (T)"() -> (w374:dbl)
                  n150 = local read "Read?"() -> (w371:bool)
                  n151 = Greater Or Equal?(x=w367, y=w368) -> (x >= y?=w370:bool)
                  n152 = Compound Arithmetic op=AND(w370, w371) -> (w369:bool)
                  n153 = case shown="False" w369 {
                    tunnel: [w377 w413] -> w372
                    tunnel: w374 -> [w375 w412]
                    tunnel: w367 -> [_ w411]
                    tunnel: w368 -> [_ w409]
                    tunnel: w373 -> [w378 w408]
                    frame True {
                      # "Ramp Up"
                      n154 = case shown="True" "First?" {
                        tunnel: [TRUE ("Save") FALSE ("Save")] -> w381
                        tunnel: [w400 w404] -> w380
                        frame False {
                          n155 = local read "Counter"() -> (w403:i8)
                          n156 = local write "Actual Polarization"(0.0 ("Actual Polarization")) -> ()
                          n157 = Increment(x=w403) -> (x+1=w400:i8)
                          n158 = local write "Counter"(w400) -> ()
                        }
                        frame True {
                          n159 = local read "Counter"() -> (w404:i8)
                          n160 = local write "First?"(FALSE ("First?")) -> ()
                        }
                      }
                      "Reset" <- w381
                      n161 = local write "Read?"(FALSE ("Read?")) -> ()
                      n162 = local read "Record ALL"() -> (w376:bool)
                      n163 = case shown="True" w376 {
                        tunnel: w380 -> [_ w388]
                        tunnel: [FALSE w386] -> w379
                        frame False {
                        }
                        frame True {
                          n164 = Greater?(x=w388, y="Max Countl") -> (0:w386:bool)
                        }
                      }
                      n165 = case shown="False" w379 {
                        tunnel: w378 -> [w392 w399]
                        tunnel: [w391 w399] -> w377
                        tunnel: w375 -> [w390 _]
                        frame False {
                          n166 = local read "Magnet"() -> (w389:bool)
                          n167 = case shown="True" w389 {
                            tunnel: w392 -> [w393 w396]
                            tunnel: [w393 w395] -> w391
                            tunnel: w390 -> [_ w394]
                            frame False {
                            }
                            frame True {
                              n168 = call "Set_B.vi"("error in (no error)"=w396, "address string"="25", "Set Field (T)"=w394) -> ("error out"=w395:errorcluster)  [unwired: 8 in]
                            }
                          }
                          "Target Field" <- w390
                        }
                        frame True {
                          "New" <- TRUE
                        }
                      }
                      "Up/Down" <- FALSE ("Up/Down")
                    }
                    frame False {
                      n169 = Less Or Equal?(x=w412, y=w409) -> (x <= y?=w410:bool)
                      n170 = case shown="False" w410 {
                        tunnel: [w414 w418] -> w413
                        tunnel: w411 -> [_ w416]
                        tunnel: w408 -> [w414 w419]
                        frame False {
                        }
                        frame True {
                          # "Resetting at the end of every cycle"
                          # "Ramp Dn"
                          n171 = local write "Up/Down"(TRUE ("Up/Down")) -> ()
                          n172 = local read "Magnet"() -> (w415:bool)
                          n173 = local write "Target Field"(w416) -> ()
                          n174 = local write "Reset"(TRUE ("Reset")) -> ()
                          n175 = case shown="True" w415 {
                            tunnel: w419 -> [w421 w424]
                            tunnel: [w421 w423] -> w418
                            tunnel: w416 -> [_ w422]
                            frame False {
                            }
                            frame True {
                              n176 = call "Set_B.vi"("error in (no error)"=w424, "address string"="25", "Set Field (T)"=w422) -> ("error out"=w423:errorcluster)  [unwired: 8 in]
                            }
                          }
                        }
                      }
                      n177 = local write "Read?"(FALSE ("Read?")) -> ()
                    }
                  }
                }
                frame True {
                  n178 = local read "Setpoint Temperature (K)"() -> (w428:dbl)
                  n179 = local read "Min Temperature (K)"() -> (w427:dbl)
                  n180 = local read "Read?"() -> (w433:bool)
                  n181 = local read "Max temperature (K)"() -> (w426:dbl)
                  n182 = Equal?(x=w428, y=w427) -> (x = y?=w431:bool)
                  n183 = And(x=w431, y=w433) -> (x .and. y?=w432:bool)
                  n184 = case shown="False" w432 {
                    tunnel: [w435 w452] -> w429
                    tunnel: w426 -> [w434 w451]
                    tunnel: w427 -> [_ w450]
                    tunnel: w428 -> [_ w448]
                    tunnel: w430 -> [w436 w447]
                    frame True {
                      # "Ramp Up"
                      n185 = local read "First?"() -> (w442:bool)
                      n186 = case shown="False" w442 {
                        frame False {
                          n187 = local read "Counter"() -> (w445:i8)
                          n188 = Increment(x=w445) -> (x+1=w444:i8)
                          n189 = local write "Counter"(w444) -> ()
                        }
                        frame True {
                        }
                      }
                      n190 = local write "Read?"(FALSE ("Read?")) -> ()
                      n191 = Number To Fractional String(number=w434, precision (6)=i16 3) -> (F-format string=w439:string)  [unwired: 2 in]
                      n192 = local read "Lake Shore"() -> (w437:refnum<visa-resource-name>)
                      n193 = Concatenate Strings("SETP 1," ("write buffer"), w439) -> (w441:string)
                      n194 = VISA Write(VISA resource name=w437, write buffer=w441, error in (no error)=w436) -> (error out=w435:errorcluster)  [unwired: 2 out]
                    }
                    frame False {
                      n195 = Equal?(x=w451, y=w448) -> (x = y?=w449:bool)
                      n196 = case shown="True" w449 {
                        tunnel: [w453 w456] -> w452
                        tunnel: w450 -> [_ w455]
                        tunnel: w447 -> [w453 w457]
                        frame False {
                        }
                        frame True {
                          # "Ramp Dn"
                          n197 = local write "Up/Down"(TRUE ("Up/Down")) -> ()
                          n198 = Number To Fractional String(number=w455, precision (6)=i16 3) -> (F-format string=w459:string)  [unwired: 2 in]
                          n199 = local read "Lake Shore"() -> (w454:refnum<visa-resource-name>)
                          n200 = Concatenate Strings("SETP 1," ("write buffer"), w459) -> (w461:string)
                          n201 = VISA Write(VISA resource name=w454, write buffer=w461, error in (no error)=w457) -> (error out=w456:errorcluster)  [unwired: 2 out]
                        }
                      }
                      n202 = local write "Read?"(FALSE ("Read?")) -> ()
                    }
                  }
                }
              }
              n203 = local read "Magnet"() -> (w353:bool)
              n204 = case shown="True" w353 {
                tunnel: [Mode."StepField" ("Enum") Mode."Plot" ("Enum")] -> w355
                frame False {
                }
                frame True {
                }
              }
            }
            frame "StepField" {
              n205 = flat-sequence {
                tunnel: w464 -> [w480]
                tunnel: [w479] -> w463
                frame #0 {
                  # "Check if it is time to step Field"
                  n206 = local read "Sweep Rate (T/min)"() -> (w481:dbl)
                  n207 = local read "B/V (T/V)"() -> (w473:dbl)
                  n208 = local read "Time Lag"() -> (w477:dbl)
                  n209 = xnode "Sweep Delay"("SweepRate"=w481, "Resolution"=0.001 ("Voltage Step (V)"), "BpV"=w473) -> ("Result"=w478:dbl)  [unwired: 1 in, 1 out]
                  n210 = Divide(x=w477, y=w478) -> (x/y=w475:dbl)
                  n211 = Multiply(x=0.001 ("y"), y=w475) -> (x*y=w474:dbl)
                  "deltaUaux" <- w474
                  n212 = stacked-sequence {
                    tunnel: w480 -> [_ w505]
                    tunnel: [_ w504] -> w479
                    tunnel: w474 -> [w483 _]
                    frame #0 {
                      n213 = local read "Actual Voltage (V)"() -> (w488:dbl)
                      n214 = local read "Up/Down"() -> (w489:bool)
                      n215 = Add(x=w488, y=w483) -> (x+y=w485:dbl)
                      n216 = Subtract(x=w488, y=w483) -> (x-y=w484:dbl)
                      n217 = Select(t=w484, s=w489, f=w485) -> (s? t:f=w487:dbl)
                      "Actual Voltage (V)" <- w487
                      n218 = local read "V/I (Ohm)"() -> (w490:dbl)
                      n219 = local read "B/V (T/V)"() -> (w491:dbl)
                      n220 = xnode "AUXtoB"("BpV"=w491, "Rm"=w490, "Aux"=w487) -> ("Result"=w486:dbl)  [unwired: 1 in, 1 out]
                      n221 = local write "Actual Field (T)"(w486) -> ()
                    }
                    frame #1 {
                      n222 = local read "Actual Voltage (V)"() -> (w510:dbl)
                      n223 = local read "Lock_in_Amplifier"() -> (w506:refnum<visa-resource-name>)
                      n224 = Format Into String(w510) -> (resulting string=w509:string)  [unwired: 3 in, 1 out]
                      n225 = Concatenate Strings("AUXV 1,", w509) -> (w507:string)
                      n226 = VISA Write(VISA resource name=w506, write buffer=w507, error in (no error)=w505) -> (error out=w504:errorcluster)  [unwired: 2 out]
                    }
                  }
                }
              }
            }
            frame "Plot" {
              # "dI"
              n227 = local read "P(uC/mm^2)"() -> (w524:dbl[])
              n228 = local read "Actual Polarization"() -> (w523:dbl)
              n229 = local read "Actual Current (pA)"() -> (w525:dbl)
              n230 = local read "Time Lag"() -> (w537:dbl)
              n231 = Multiply(x=w525, y=w537) -> (x*y=w529:dbl)
              n232 = Divide(x=w529, y="Sample area (mm^2)") -> (x/y=w528:dbl)
              n233 = Add(x=w528, y=w523) -> (x+y=w527:dbl)
              "Actual Polarization" <- w527
              n234 = local read "Temp/Magnetic Field"() -> (w538:bool)
              n235 = Build Array (concatenate)(w524, w527) -> (→"P(uC/mm^2)":dbl[])
              n236 = case shown="False" w538 {
                tunnel: w535 -> [_ w606]
                tunnel: w532 -> [_ w588]
                tunnel: w527 -> [w545 w589]
                frame False {
                  # "Magnetic Field plotting"
                  n237 = local read "Up/Down"() -> (w550:bool)
                  n238 = case shown="True" w550 {
                    frame True {
                      # "Down"
                      n239 = local read "I(B) 3"() -> (w560:cluster{dbl[], dbl[]}[])
                      n240 = local read "I(B) 3"() -> (w564:cluster{dbl[], dbl[]}[])
                      n241 = Index Array(array=w560, index=1) -> (element=w558:cluster{dbl[], dbl[]})
                      n242 = Unbundle(w558) -> (w557:dbl[], w556:dbl[])
                      n243 = Index Array(array=w564, index=i8 0 ("t")) -> (element=w561:cluster{dbl[], dbl[]})
                      n244 = local read "Actual Current (pA)"() -> (w551:dbl)
                      n245 = local read "Actual B Field (T)"() -> (w553:dbl)
                      n246 = Build Array (concatenate)(w557, w553) -> (w555:dbl[])
                      n247 = Build Array (concatenate)(w556, w551) -> (w554:dbl[])
                      n248 = Bundle(w555, w554) -> (w552:cluster{dbl[], dbl[]})  [unwired: 1 in]
                      n249 = Build Array(w561, w552) -> (w562:cluster{dbl[], dbl[]}[])
                      n250 = local write "I(B) 3"(w562) -> ()
                    }
                    frame False {
                      # "Up"
                      n251 = local read "I(B) 3"() -> (w576:cluster{dbl[], dbl[]}[])
                      n252 = local read "I(B) 3"() -> (w578:cluster{dbl[], dbl[]}[])
                      n253 = Index Array(array=w576, index=0) -> (element=w574:cluster{dbl[], dbl[]})
                      n254 = Unbundle(w574) -> (w573:dbl[], w572:dbl[])
                      n255 = Index Array(array=w578, index=i8 1 ("t")) -> (element=w567:cluster{dbl[], dbl[]})
                      n256 = local read "Actual B Field (T)"() -> (w568:dbl)
                      n257 = Build Array (concatenate)(w573, w568) -> (w571:dbl[])
                      n258 = local read "Actual Current (pA)"() -> (w565:dbl)
                      n259 = Build Array (concatenate)(w572, w565) -> (w570:dbl[])
                      n260 = Bundle(w571, w570) -> (w569:cluster{dbl[], dbl[]})  [unwired: 1 in]
                      n261 = Build Array(w569, w567) -> (w566:cluster{dbl[], dbl[]}[])
                      n262 = local write "I(B) 3"(w566) -> ()
                    }
                  }
                  n263 = local read "Actual B Field (T)"() -> (w547:dbl)
                  n264 = local read "P(B)"() -> (w549:cluster{"yi":dbl[], dbl[]})
                  n265 = Unbundle(w549) -> ("yi"=w548:dbl[], w546:dbl[])
                  n266 = Build Array (concatenate)(w548, w547) -> (w544:dbl[])
                  n267 = Build Array (concatenate)(w546, w545) -> (w543:dbl[])
                  n268 = Bundle(w544, w543) -> (→"P(B)":cluster{dbl[], dbl[]})  [unwired: 1 in]
                }
                frame True {
                  # "Temperature plotting"
                  n269 = Quotient & Remainder(x=w606, y="Save Period") -> (x-y*floor(x/y)=w587:dbl)  [unwired: 1 out]
                  n270 = Greater?(x=w588, y=w587) -> (0:w604:bool)
                  n271 = local read "MagnetoResistance (Ohm)"() -> (w586:cluster{dbl[], dbl[]})
                  n272 = local read "Actual Temperature (K)"() -> (w584:dbl)
                  n273 = local read "Actual Temperature (K)"() -> (w591:dbl)
                  n274 = local read "Actual Current (pA)"() -> (w597:dbl)
                  n275 = local read "MagnetoRes (Ohm)"() -> (w582:dbl)
                  n276 = local read "P(T)"() -> (w593:cluster{"yi":dbl[], dbl[]})
                  n277 = local read "I(T)"() -> (w603:cluster{dbl[], dbl[]})
                  n278 = case shown="True" w604 {
                    frame False {
                    }
                    frame True {
                      n279 = local write "Reset"(TRUE) -> ()
                    }
                  }
                  n280 = Unbundle(w593) -> ("yi"=w594:dbl[], w590:dbl[])
                  n281 = Unbundle(w603) -> (w601:dbl[], w600:dbl[])
                  n282 = Unbundle(w586) -> (w585:dbl[], w583:dbl[])
                  n283 = Build Array (concatenate)(w594, w591) -> (w595:dbl[])
                  n284 = Build Array (concatenate)(w590, w589) -> (w596:dbl[])
                  n285 = Build Array (concatenate)(w585, w584) -> (w581:dbl[])
                  n286 = Build Array (concatenate)(w601, w591) -> (w599:dbl[])
                  n287 = Build Array (concatenate)(w600, w597) -> (w598:dbl[])
                  n288 = Build Array (concatenate)(w583, w582) -> (w580:dbl[])
                  n289 = Bundle(w599, w598) -> (→"I(T)":cluster{dbl[], dbl[]})  [unwired: 1 in]
                  n290 = Bundle(w581, w580) -> (→"MagnetoResistance (Ohm)":cluster{dbl[], dbl[]})  [unwired: 1 in]
                  n291 = Bundle(w595, w596) -> (→"P(T)":cluster{dbl[], dbl[]})  [unwired: 1 in]
                }
              }
            }
            frame "Save" {
              n292 = local read "Reset"() -> (w608:bool)
              n293 = case shown="True" w608 {
                tunnel: w613 -> [w630 w632]
                tunnel: [w630 w635] -> w618
                tunnel: w612 -> [w629 w633]
                tunnel: [w629 w635] -> w617
                tunnel: w614 -> [w628 w634]
                tunnel: [w628 w635] -> w616
                tunnel: [w627 w635] -> w615
                tunnel: w611 -> [w627 w631]
                frame False {
                }
                frame True {
                  n294 = stacked-sequence {
                    tunnel: [_ _ w685] -> w635
                    tunnel: w634 -> [_ w674 _]
                    tunnel: w633 -> [w659 w672 _]
                    tunnel: w632 -> [w660 w673 _]
                    tunnel: w631 -> [w649 w670 _]
                    frame #0 {
                      n295 = local read "B array"() -> (w642:dbl[])
                      n296 = local read "Counter"() -> (w658:i8)
                      n297 = local read "Averaged I(B)"() -> (w662:dbl[][])
                      n298 = local read "Up/Down"() -> (w661:bool)
                      n299 = local read "Sample area (mm^2)"() -> (w638:dbl)
                      n300 = call "Average_IBP_curves.vi"("I in"=w659, "Averaged P(B) In"="Averaged P(B)", "Counter"=w658, "Averaged I(B) In"=w662, "t in"=w649, "B in"=w660, "Averaged dt in"="Averaged dt", "Up/Down"=w661, "Sample area(mm^2)"=w638, "B array"=w642) -> ("Averaged I(B) out"=w653:dbl[][], "Averaged dt Out"=w646:dbl[][], "Averaged P(B) Out"=w645:dbl[][])  [unwired: 3 in]
                      "Averaged I(B)" <- w653
                      n301 = Index Array(array=w645, index (row)=0 ("disabled index (col)")) -> (element=w643:dbl[])  [unwired: 1 in]
                      n302 = Index Array(array=w645, index (row)=1 ("disabled index (col)")) -> (element=w644:dbl[])  [unwired: 1 in]
                      n303 = local write "Averaged P(B)"(w645) -> ()
                      n304 = Index Array(array=w653, index (row)=0 ("disabled index (col)")) -> (element=w651:dbl[])  [unwired: 1 in]
                      n305 = Index Array(array=w653, index (row)=1 ("disabled index (col)")) -> (element=w650:dbl[])  [unwired: 1 in]
                      n306 = local write "Averaged dt"(w646) -> ()
                      n307 = Bundle("B array"=w642, "Averaged P(B) Out"=w643) -> (w641:T7)  [unwired: 1 in]
                      n308 = Bundle("B array"=w642, "Averaged P(B) Out"=w644) -> (w640:T7)  [unwired: 1 in]
                      n309 = Bundle("B array"=w642, "Averaged I(B) out"=w651) -> (w657:T8)  [unwired: 1 in]
                      n310 = Bundle("B array"=w642, "Averaged I(B) out"=w650) -> (w656:T8)  [unwired: 1 in]
                      n311 = Build Array(w641, w640) -> (→"P(B) /Averaged/":T9)
                      n312 = Build Array(w657, w656) -> (→"I(B) /Averaged/":T10)
                    }
                    frame #1 {
                      # "Save and Reset"
                      n313 = local read "Temp/Magnetic Field"() -> (w663:bool)
                      n314 = local read "Measurement File"() -> (w665:path)
                      n315 = local read "P(uC/mm^2)"() -> (w671:dbl[])
                      n316 = Build Array(w674, w673, w672, w670, w671) -> (w664:dbl[][])
                      n317 = case shown="False" w663 {
                        tunnel: w665 -> [_ _]
                        tunnel: w664 -> [w679 _]
                        frame False {
                          n318 = local read "Up/Down"() -> (w677:bool)
                          n319 = case shown="False" w677 {
                            tunnel: [w682 w683] -> w676
                            frame False {
                              n320 = local read "Measurement File_dn"() -> (w682:path)
                            }
                            frame True {
                              n321 = local read "Measurement File_up"() -> (w683:path)
                            }
                          }
                          n322 = call-poly <vilib>:"Write Delimited Spreadsheet.vi"("file path (dialog if empty)"=w676, "format (%.3f)"="%.5g", "2D data"=w679, "append to file? (F)"=TRUE ("transpose? (F)"), "transpose? (F)"=FALSE ("append to file? (F)")) -> ()  [unwired: 9 in, 2 out]
                        }
                        frame True {
                        }
                      }
                      n323 = case shown="False" "Reset IB?" {
                        frame False {
                        }
                        frame True {
                          n324 = local read "Up/Down"() -> (w684:bool)
                          n325 = case shown="False" w684 {
                            frame False {
                              n326 = invoke on="I(B) 3" class="XYGraph (strict)" method="Reinit To Default"() -> ()  [unwired: 3 in, 3 out]
                            }
                            frame True {
                            }
                          }
                        }
                      }
                      n327 = call-poly <vilib>:"Write Delimited Spreadsheet.vi"("file path (dialog if empty)"=w665, "format (%.3f)"="%.5g", "2D data"=w664, "append to file? (F)"=TRUE, "transpose? (F)"=TRUE) -> ()  [unwired: 9 in, 2 out]
                      n328 = local write "Reset"(FALSE ("Save")) -> ()
                    }
                    frame #2 {
                      w685 = dbl[] []
                      n329 = local write "P(uC/mm^2)"(w685) -> ()
                    }
                  }
                }
              }
              n330 = local read "New"() -> (w610:bool)
              n331 = case shown="True" w610 {
                tunnel: [Mode."Return" ("Enum") Mode."New" ("Enum")] -> w622
                tunnel: [TRUE FALSE] -> w609
                frame False {
                }
                frame True {
                }
              }
            }
            frame "New" {
              n332 = stacked-sequence {
                seq-local: [_ _ _ _ w779 _ _] -> [_ _ _ _ _ w788 _]
                seq-local: [_ _ w733 _ _ _ _] -> [_ _ _ _ w778 _ _]
                tunnel: T6 {"Com Port"=1, "ISOBUS Address"=0, "GPIB Address"=25, "Communication"=enum."GPIB"} ("Address") -> [_ _ w732 w773 _ _ _]
                tunnel: w688 -> [_ _ w734 _ _ w789 _]
                tunnel: [_ _ _ _ _ w791 _] -> w687
                tunnel: w686 -> [_ w713 _ _ _ _ _]
                frame #0 {
                  # "Save averages"
                  n333 = local read "Measurement File_average"() -> (w701:path)
                  n334 = local read "I(B) /Averaged/"() -> (w702:cluster{"B array":dbl[], dbl[]}[])
                  n335 = Index Array(array=w702, index=0) -> (element=w705:cluster{"B array":dbl[], dbl[]})
                  n336 = Index Array(array=w702, index=1) -> (element=w706:cluster{"B array":dbl[], dbl[]})
                  n337 = Unbundle(w705) -> ("B array"=w707:dbl[], w708:dbl[])
                  n338 = Unbundle(w706) -> ("B array"=w709:dbl[], w710:dbl[])
                  n339 = Build Array(w707, w708, w709, w710) -> (w711:dbl[][])
                  n340 = call-poly <vilib>:"Write Delimited Spreadsheet.vi"("file path (dialog if empty)"=w701, "format (%.3f)"="%.5g", "2D data"=w711, "append to file? (F)"=TRUE ("transpose? (F)"), "transpose? (F)"=TRUE ("append to file? (F)")) -> ()  [unwired: 9 in, 2 out]
                }
                frame #1 {
                  w719 = dbl[] []
                  w728 = dbl[] []
                  # "Reset Flags"
                  n341 = Get Date/Time In Seconds() -> (seconds since 1Jan1904=w729:timestamp)
                  n342 = local write "Up/Down"(TRUE ("Up/Down")) -> ()
                  n343 = local write "First?"(TRUE ("First?")) -> ()
                  n344 = local write "Offset?"(FALSE ("Offset?")) -> ()
                  n345 = local write "New"(FALSE ("New")) -> ()
                  n346 = local write "P(uC/mm^2)"(w728) -> ()
                  n347 = local write "Start time"(w729) -> ()
                  n348 = local write "Offset array"(w728) -> ()
                  n349 = local write "Actual Polarization"(0.0 ("Actual Polarization")) -> ()
                  n350 = local write "Up/Down"(TRUE ("Up/Down")) -> ()
                  n351 = local write "Reset"(FALSE ("Reset")) -> ()
                  n352 = local read "B array"() -> (w722:dbl[])
                  n353 = local write "Counter"(i8 0 ("Counter")) -> ()
                  n354 = invoke on="P(B)" class="XYGraph (strict)" method="Reinit To Default"() -> ()  [unwired: 3 in, 3 out]
                  n355 = invoke on="I(B) 3" class="XYGraph (strict)" method="Reinit To Default"() -> ()  [unwired: 3 in, 3 out]
                  n356 = Multiply(x=w722, y=0.0) -> (x*y=w723:dbl[])
                  n357 = Build Array(w719, w719) -> (w727:dbl[][])
                  n358 = Bundle("B array"=w722, w723) -> (w724:cluster{"B array":dbl[], dbl[]})  [unwired: 1 in]
                  n359 = local write "Averaged I(B)"(w727) -> ()
                  n360 = Build Array(w724, w724) -> (w725:cluster{"B array":dbl[], dbl[]}[])
                  n361 = local write "I(B) /Averaged/"(w725) -> ()
                  n362 = local write "Measuring"(FALSE ("Measuring")) -> ()
                  n363 = Flush Queue(queue=w713) -> (remaining elements=→"remaining elements":T1)  [unwired: 1 in, 2 out]
                }
                frame #2 {
                  # "Step"
                  n364 = local read "Sweep Rate Array"() -> (w738:dbl[])
                  n365 = local read "j"() -> (w739:i32)
                  n366 = Increment(x=w739) -> (x+1=w735:i32)
                  n367 = Array Size(array=w738) -> (size(s)=w737:i32)
                  n368 = Less?(x=w735, y=w737) -> (x < y?=w736:bool)
                  "Step Rate" <- w736
                  n369 = case shown="True" w736 {
                    tunnel: w735 -> [_ w766]
                    tunnel: w734 -> [w742 w765]
                    tunnel: [w741 w765] -> w733
                    tunnel: w732 -> [w740 _]
                    frame False {
                      # "Step Temp?"
                      n370 = local read "Temperature Array"() -> (w746:dbl[])
                      n371 = local read "i"() -> (w747:i32)
                      n372 = Increment(x=w747) -> (x+1=w744:i32)
                      n373 = local write "j"(0 ("f")) -> ()
                      n374 = Array Size(array=w746) -> (size(s)=w745:i32)
                      n375 = Less?(x=w744, y=w745) -> (x < y?=w743:bool)
                      "Step Temp" <- w743
                      n376 = case shown="False" w743 {
                        tunnel: w744 -> [_ w764]
                        tunnel: w742 -> [w752 w763]
                        tunnel: [w751 w763] -> w741
                        tunnel: w740 -> [w750 _]
                        frame False {
                          # "Heater OFF"
                          # "Finished"
                          n377 = local write "i"(0 ("i")) -> ()
                          n378 = stacked-sequence {
                            tunnel: w752 -> [w756 _ _]
                            tunnel: [w755 _ _] -> w751
                            tunnel: w750 -> [_ w760 w761]
                            frame #0 {
                              n379 = local read "Lake Shore"() -> (w757:refnum<visa-resource-name>)
                              n380 = VISA Write(VISA resource name=w757, write buffer="RANGE,1,0", error in (no error)=w756) -> (error out=w755:errorcluster)  [unwired: 2 out]
                            }
                            frame #1 {
                              n381 = call "ips_switchHeaterOff.vi"("Instrument address"=w760, "Rate"=2.0) -> ()  [unwired: 1 out]
                            }
                            frame #2 {
                              n382 = call "GPIB - BusCommand.vi"("Command"="H0", "Address"=w761) -> ()  [unwired: 2 out]
                            }
                          }
                          n383 = local write "Record ALL"(FALSE ("Record ALL")) -> ()
                          "Finished" <- TRUE
                        }
                        frame True {
                          n384 = local write "i"(w764) -> ()
                        }
                      }
                    }
                    frame True {
                      n385 = local write "j"(w766) -> ()
                    }
                  }
                }
                frame #3 {
                  # "Set rates"
                  n386 = local read "Sweep Rate Array"() -> (w772:dbl[])
                  n387 = local read "j"() -> (w771:i32)
                  n388 = local read "j"() -> (w769:i32)
                  n389 = Index Array(array=w772, index=w771) -> (element=w770:dbl)
                  n390 = Number To Fractional String(number=w770, precision (6)=i16 3) -> (F-format string=w776:string)  [unwired: 2 in]
                  n391 = Index Array(array="Max count array", index=w769) -> (element=w767:i32)
                  n392 = local write "Max Countl"(w767) -> ()
                  n393 = Concatenate Strings("T" ("format string"), w776) -> (w777:string)
                  n394 = call "GPIB - BusCommand.vi"("Command"=w777, "Address"=w773) -> ()  [unwired: 2 out]
                  n395 = local write "Sweep Rate (T/min)"(w770) -> ()
                }
                frame #4 {
                  # "Set temperature"
                  n396 = local read "Temperature Array"() -> (w782:dbl[])
                  n397 = local read "i"() -> (w781:i32)
                  n398 = Index Array(array=w782, index=w781) -> (element=w780:dbl)
                  n399 = local read "Lake Shore"() -> (w784:refnum<visa-resource-name>)
                  n400 = Number To Fractional String(number=w780, precision (6)=i16 3) -> (F-format string=w785:string)  [unwired: 2 in]
                  n401 = Concatenate Strings("SETP 1," ("write buffer"), w785) -> (w787:string)
                  n402 = VISA Write(VISA resource name=w784, write buffer=w787, error in (no error)=w778) -> (error out=w779:errorcluster)  [unwired: 2 out]
                }
                frame #5 {
                  n403 = local read "Finished"() -> (w790:bool)
                  n404 = case shown="False" w790 {
                    tunnel: [w804 w841] -> w791
                    tunnel: w789 -> [_ _]
                    tunnel: w788 -> [w801 w841]
                    frame False {
                      w799 = "_" ("string")
                      # "Wait, create Files"
                      n405 = local read "Temperature Array"() -> (w831:dbl[])
                      n406 = local read "Sweep Rate Array"() -> (w827:dbl[])
                      n407 = local read "i"() -> (w830:i32)
                      n408 = local read "j"() -> (w828:i32)
                      n409 = Index Array(array=w831, index=w830) -> (element=w829:dbl)
                      n410 = Index Array(array=w827, index=w828) -> (element=w796:dbl)
                      n411 = Round Toward -Infinity(1:w796) -> (0:w797:dbl)
                      n412 = Number To Fractional String(use system decimal point (T)=TRUE, number=w829, precision (6)=i16 1) -> (F-format string=w832:string)  [unwired: 1 in]
                      n413 = Subtract(x=w796, y=w797) -> (x-y=w798:dbl)
                      n414 = Equal To 0?(x=w798) -> (x = 0?=w795:bool)
                      n415 = Select(t=i16 0 ("precision (6)"), s=w795, f=i16 2 ("precision (6)")) -> (s? t:f=w792:i16)
                      n416 = Number To Fractional String(use system decimal point (T)=TRUE, number=w796, precision (6)=w792) -> (F-format string=w800:string)  [unwired: 1 in]
                      n417 = Concatenate Strings("Directory", "\\" ("string"), "FileName", w799, w832, "K" ("string"), w799, w800, "Tpm" ("string")) -> (w821:string)
                      n418 = Search and Replace String(replace all?=TRUE ("replace all? (F)"), input string=w821, search string=".", replace string="p" ("substring (\"\")"), error in=w801) -> (result string=w816:string, error out=w811:errorcluster)  [unwired: 3 in, 2 out]
                      n419 = local write "Step Rate"(FALSE ("Step Rate")) -> ()
                      n420 = Concatenate Strings(w816, ".txt" ("string")) -> (w815:string)
                      n421 = local read "Step Temp"() -> (w805:bool)
                      n422 = String To Path(string=w815) -> (path=w814:path)
                      n423 = Open/Create/Replace File(file path (use dialog)=w814, error in=w811, operation (0:open)=T5."open or create") -> (refnum out=w803:refnum<file>, error out=w804:errorcluster)  [unwired: 3 in, 1 out]
                      n424 = local write "refnum out"(w803) -> ()
                      n425 = Refnum to Path(1:w803) -> (0:w806:path)
                      n426 = call "Create_sweep_files.vi"("Measurement File"=w806) -> ("Path 3"=w809:path, "Path 2"=w808:path, "Path"=w807:path)  [unwired: 8 in]
                      n427 = local write "Measurement File"(w806) -> ()
                      n428 = case shown="True" w805 {
                        frame False {
                        }
                        frame True {
                          n429 = Get Date/Time In Seconds() -> (seconds since 1Jan1904=w834:timestamp)
                          n430 = local write "Step Temp"(FALSE ("Step Temp")) -> ()
                          n431 = while {
                            tunnel: w834 -> [w839]
                            stop <- w836 stop-if-true
                            n432 = Get Date/Time In Seconds() -> (seconds since 1Jan1904=w840:timestamp)
                            n433 = Subtract(x=w840, y=w839) -> (x-y=w838:dbl)
                            "Wait (s)" <- w838
                            n434 = Greater Or Equal?(x=w838, y="secs to wait") -> (x >= y?=w836:bool)
                          }
                        }
                      }
                      n435 = local write "Measurement File_dn"(w809) -> ()
                      n436 = local write "Measurement File_average"(w807) -> ()
                      n437 = local write "Measurement File_up"(w808) -> ()
                    }
                    frame True {
                    }
                  }
                }
                frame #6 {
                  n438 = local read "Finished"() -> (w842:bool)
                  n439 = case shown="True" w842 {
                    frame False {
                      n440 = local write "Measuring"(TRUE ("Measuring")) -> ()
                    }
                    frame True {
                      n441 = local write "Measure /Pause"(FALSE ("Measure /Pause")) -> ()
                    }
                  }
                }
              }
            }
            frame "Return" {
            }
          }
        }
      }
      frame Error {
        # "Return true for any case which should stop the loop."
      }
    }
  }
  n442 = case shown="True" w49 {
    frame False {
    }
    frame True {
      n443 = invoke on="P(T)" class="XYGraph (strict)" method="Reinit To Default"() -> ()  [unwired: 3 in, 3 out]
      n444 = invoke on="I(T)" class="XYGraph (strict)" method="Reinit To Default"() -> ()  [unwired: 3 in, 3 out]
    }
  }
  n445 = while {
    shift-right: [w874] -> w88
    shift-left: w69 -> [w875]
    shift-right: [w876] -> w95
    shift-left: w96 -> [w877]
    tunnel: w91 -> [w873]
    tunnel: w90 -> [w872]
    tunnel: w35 -> [w871]
    tunnel: [w865] -> _
    tunnel: w77 -> [w864]
    tunnel: w67 -> [w863]
    tunnel: w11 -> [w862]
    stop <- "stop" stop-if-true
    n446 = event shown="[0] Timeout" {
      selector: _ -> [_ _ _ _ _ _ _ _ _ _ _ _ _ _ _]
      dyn-events: _ -> [_ _ _ _ _ _ _ _ _ _ _ _ _ _ _]
      timeout: 10 -> [_ _ _ _ _ _ _ _ _ _ _ _ _ _ _]
      tunnel: w877 -> [w888 w925 w935 w949 w1020 w1024 w1028 w1060 w1076 w1093 w1136 w1153 w1169 w1179 w1190]
      tunnel: [w887 w925 w935 w949 w1020 w1024 w1028 w1060 w1076 w1093 w1136 w1153 w1169 w1179 w1190] -> w876
      tunnel: w875 -> [w886 w924 w934 w947 w1019 w1026 w1030 w1061 w1075 w1092 w1137 w1155 w1173 w1183 w1192]
      tunnel: [w885 w924 w934 w946 w1021 w1026 w1029 _ w1075 w1092 w1137 w1154 w1172 w1182 w1191] -> w874
      tunnel: w873 -> [w884 _ _ _ _ _ _ _ _ _ _ _ _ _ _]
      tunnel: w872 -> [w883 _ _ _ _ _ _ _ _ _ _ _ _ _ _]
      tunnel: w871 -> [w882 _ _ _ _ _ _ _ _ _ _ _ _ _ _]
      tunnel: [w880 w923 w933 w948 w1022 w1025 w1027 w1059 w1074 w1091 w1135 w1152 w1170 w1180 _] -> w865
      tunnel: w864 -> [w880 w923 w936 w948 w1022 w1025 w1027 w1059 w1074 w1091 w1135 w1152 w1170 w1180 _]
      tunnel: w863 -> [_ _ _ _ _ _ _ _ _ _ _ w1156 w1171 w1184 w1189]
      tunnel: [_ _ _ _ _ _ _ w1061 _ _ _ _ _ _ _] -> _
      tunnel: w862 -> [w879 _ _ _ _ _ _ _ _ _ _ _ _ _ _]
      event Timeout {
        n447 = event-data() -> ()  [unwired: 1 in, 3 out]
        n448 = case shown="True" "Measuring" {
          tunnel: w888 -> [w890 w914]
          tunnel: [w890 w913] -> w887
          tunnel: w886 -> [w889 _]
          tunnel: [w889 w912] -> w885
          tunnel: w884 -> [_ w905]
          tunnel: w883 -> [_ w904]
          tunnel: w882 -> [_ w900]
          tunnel: w879 -> [_ w896]
          frame False {
          }
          frame True {
            w903 = ":FETCh? " ("data")
            w906 = u32 1000 ("byte count")
            # "Generate the data here."
            n449 = local read "Number of Samples"() -> (w891:i32)
            n450 = case shown="No Error" w900 {
              selector: w900 -> [w916 w917]
              tunnel: [w916 w917] -> w899
              tunnel: [w915 _] -> w898
              frame No Error {
                n451 = Get Date/Time In Seconds() -> (seconds since 1Jan1904=w915:timestamp)
              }
              frame Error {
              }
            }
            n452 = VISA Write(VISA resource name=w905, write buffer=w903, error in (no error)=w899) -> (VISA resource name out=w911:refnum<visa-resource-name>, error out=w909:errorcluster)  [unwired: 1 out]
            n453 = VISA Write(VISA resource name=w904, write buffer=w903, error in (no error)=w909) -> (VISA resource name out=w910:refnum<visa-resource-name>, error out=w908:errorcluster)  [unwired: 1 out]
            n454 = VISA Read(VISA resource name=w911, byte count=w906, error in (no error)=w908) -> (read buffer=w901:string, error out=w907:errorcluster)  [unwired: 2 out]
            n455 = VISA Read(VISA resource name=w910, byte count=w906, error in (no error)=w907) -> (read buffer=w902:string, error out=w895:errorcluster)  [unwired: 2 out]
            n456 = call-poly <vilib>:"DAQmx Read.vi"("task/channels in"=w896, "number of samples per channel"=w891, "error in"=w895) -> ("data"=w893:dbl[], "error out"=w894:errorcluster)  [unwired: 10 in, 1 out]
            n457 = call-poly <vilib>:"Mean.vi"("X"=w893) -> ("mean"=w892:dbl)  [unwired: 1 out]
            "mean" <- w892
            n458 = Bundle("seconds since 1Jan1904"=w898, "read buffer"=w901, "read buffer"=w902, "mean"=w892) -> (w897:T4)  [unwired: 1 in]
            n459 = Enqueue Element(queue=w914, element=w897, error in (no error)=w894) -> (queue out=w913:refnum<queue>, error out=w912:errorcluster)  [unwired: 1 in, 1 out]
          }
        }
      }
      event "Max Field (T)": Value Change {
        n460 = event-data() -> ()  [unwired: 1 in, 6 out]
        n461 = Divide(x="Max Field (T)", y="dB (T)") -> (x/y=w920:dbl)
        n462 = for {
          N: w920 -> [_]
          tunnel: "dB (T)" -> [w930]
          tunnel: [w927] -> w919 mode=indexing
          tunnel: "Min Field (T)" -> [w928]
          tunnel: [0.0] -> _ mode=indexing
          i -> [w931]
          n463 = Multiply(x=w931, y=w930) -> (x*y=w929:dbl)
          n464 = Add(x=w929, y=w928) -> (x+y=w927:dbl)
        }
        "B array" <- w919
      }
      event "Sweep Rate (T/min)": Value Change {
        n465 = event-data() -> ("NewVal"=w937:dbl)  [unwired: 1 in, 5 out]
        n466 = local read "Magnet"() -> (w932:bool)
        n467 = case shown="False" w932 {
          tunnel: w937 -> [_ w944]
          tunnel: w936 -> [w938 w940]
          tunnel: [w938 w939] -> w933
          frame False {
          }
          frame True {
            n468 = Number To Fractional String(number=w944, precision (6)=i16 3) -> (F-format string=w942:string)  [unwired: 2 in]
            n469 = Concatenate Strings("T" ("format string"), w942) -> (w941:string)
            n470 = call "GPIB - BusCommand.vi"("Command"=w941, "Address"=w940) -> ("Address(thru)"=w939:T6)  [unwired: 1 out]
          }
        }
      }
      event "Field To Zero": Value Change {
        n471 = event-data() -> ()  [unwired: 1 in, 6 out]
        n472 = Two Button Dialog(message="Do you want to switch off the field?", 1:"No" ("F button name (\"Cancel\")"), 2:"Yes" ("T button name (\"OK\")")) -> (T button?=w953:bool)
        n473 = case shown="True" w953 {
          tunnel: w948 -> [_ w958]
          tunnel: w947 -> [w954 w956]
          tunnel: [w954 w955] -> w946
          frame False {
          }
          frame True {
            n474 = local read "Magnet"() -> (w957:bool)
            n475 = case shown="False" w957 {
              tunnel: w958 -> [_ w1010]
              tunnel: w956 -> [w961 w1007]
              tunnel: [w960 w1007] -> w955
              frame False {
                n476 = local read "Lock_in_Amplifier"() -> (w959:refnum<visa-resource-name>)
                n477 = stacked-sequence {
                  seq-local: [w964 _] -> [_ w976]
                  seq-local: [w962 _] -> [_ w973]
                  tunnel: w961 -> [w966 _]
                  tunnel: [_ w979] -> w960
                  tunnel: w959 -> [w963 w974]
                  frame #0 {
                    n478 = VISA Write(VISA resource name=w963, write buffer="AUXV?1", error in (no error)=w966) -> (VISA resource name out=w970:refnum<visa-resource-name>, error out=w965:errorcluster)  [unwired: 1 out]
                    n479 = VISA Read(VISA resource name=w970, byte count=u32 1000, error in (no error)=w965) -> (read buffer=w967:string, error out=w964:errorcluster)  [unwired: 2 out]
                    n480 = Fract/Exp String To Number(string=w967) -> (number=w962:dbl)  [unwired: 3 in, 1 out]
                  }
                  frame #1 {
                    w982 = 0.001 ("Voltage Step (V)")
                    n481 = local read "Sweep Rate (T/min)"() -> (w981:dbl)
                    n482 = local read "V/I (Ohm)"() -> (w978:dbl)
                    n483 = local read "B/V (T/V)"() -> (w972:dbl)
                    n484 = xnode "Sweep Delay"("SweepRate"=w981, "Resolution"=w982, "BpV"=w972) -> ("Result"=w980:dbl)  [unwired: 1 in, 1 out]
                    n485 = call "Universal_Ramping.vi"("milliseconds to wait"=w980, "Initial Voltage (V)"=w973, "error in (no error)"=w976, "Voltage Step (V)"=w982, "Final Voltage (V)"=0.0, "VISA resource name"=w974) -> ("error out"=w979:errorcluster, "Actual Voltage (V)"=w971:dbl)  [unwired: 3 in, 1 out]
                    n486 = local write "Actual Voltage (V)"(w971) -> ()
                    n487 = xnode "AUXtoB"("BpV"=w972, "Rm"=w978, "Aux"=w971) -> ("Result"=w977:dbl)  [unwired: 1 in, 1 out]
                    n488 = local write "Actual B Field (T)"(w977) -> ()
                  }
                }
              }
              frame True {
                n489 = local read "Sweep Rate (T/min)"() -> (w1009:dbl)
                n490 = call "ips_switchHeaterOff.vi"("Instrument address"=w1010, "Rate"=w1009) -> ("B"=w1008:dbl)
                n491 = local write "Actual Field (T)"(w1008) -> ()
              }
            }
          }
        }
      }
      event "Go to Set": Value Change {
        n492 = event-data() -> ()  [unwired: 1 in, 6 out]
        n493 = local read "V/I (Ohm)"() -> (w1017:dbl)
        n494 = local read "B/V (T/V)"() -> (w1016:dbl)
        n495 = local read "Lock_in_Amplifier"() -> (w1013:refnum<visa-resource-name>)
        n496 = local read "Sweep Rate (T/min)"() -> (w1015:dbl)
        n497 = local read "Magnet"() -> (w1018:bool)
        n498 = call "Ramp_Field.vi"("Set Field (T) in"="Set Field (T)", "Sweep Rate (T/min)"=w1015, "V/I (Ohm)"=w1017, "error in (no error)"=w1019, "Magnet"=w1018, "B/V (T/V)"=w1016, "VISA Refnum in"=w1013) -> ("error out"=w1021:errorcluster, "Actual Voltage (V)"=w1011:dbl, "Set Field (T) out"=w1014:dbl)  [unwired: 2 in]
        n499 = local write "Actual B Field (T)"(w1014) -> ()
        n500 = local write "Actual Voltage (V)"(w1011) -> ()
      }
      event "Measure /Pause": Value Change {
        n501 = event-data() -> ("NewVal"=w1023:bool)  [unwired: 1 in, 5 out]
        n502 = local write "Measuring"(w1023) -> ()
      }
      event "Stop": Value Change {
        n503 = event-data() -> ()  [unwired: 1 in, 6 out]
        n504 = local read "Measuring"() -> (w1031:bool)
        n505 = case shown="True" w1031 {
          tunnel: w1030 -> [w1032 w1035]
          tunnel: [w1032 w1036] -> w1029
          frame False {
          }
          frame True {
            w1043 = FALSE ("Measuring")
            n506 = local read "SaveSweep"() -> (w1044:bool)
            n507 = local write "Measuring"(w1043) -> ()
            n508 = local write "Measure /Pause"(w1043) -> ()
            n509 = local read "Lock_in_Amplifier"() -> (w1037:refnum<visa-resource-name>)
            n510 = case shown="True" w1044 {
              frame False {
              }
              frame True {
                n511 = local read "Measurement File_average"() -> (w1055:path)
                n512 = local read "I(B) /Averaged/"() -> (w1054:cluster{"B array":dbl[], dbl[]}[])
                n513 = Index Array(array=w1054, index=0) -> (element=w1051:cluster{"B array":dbl[], dbl[]})
                n514 = Index Array(array=w1054, index=1) -> (element=w1050:cluster{"B array":dbl[], dbl[]})
                n515 = Unbundle(w1051) -> ("B array"=w1049:dbl[], w1048:dbl[])
                n516 = Unbundle(w1050) -> ("B array"=w1047:dbl[], w1046:dbl[])
                n517 = Build Array(w1049, w1048, w1047, w1046) -> (w1045:dbl[][])
                n518 = call-poly <vilib>:"Write Delimited Spreadsheet.vi"("file path (dialog if empty)"=w1055, "format (%.3f)"="%.5g", "2D data"=w1045, "append to file? (F)"=TRUE ("transpose? (F)"), "transpose? (F)"=TRUE ("append to file? (F)")) -> ()  [unwired: 9 in, 2 out]
              }
            }
            n519 = local read "V/I (Ohm)"() -> (w1041:dbl)
            n520 = local read "Sweep Rate (T/min)"() -> (w1040:dbl)
            n521 = local read "Set Field (T)"() -> (w1042:dbl)
            n522 = local read "B/V (T/V)"() -> (w1038:dbl)
            n523 = local read "Magnet"() -> (w1039:bool)
            n524 = call "Ramp_Field.vi"("Set Field (T) in"=w1042, "Sweep Rate (T/min)"=w1040, "V/I (Ohm)"=w1041, "error in (no error)"=w1035, "Magnet"=w1039, "B/V (T/V)"=w1038, "VISA Refnum in"=w1037) -> ("error out"=w1036:errorcluster, "Actual Voltage (V)"=w1033:dbl, "Set Field (T) out"=w1034:dbl)  [unwired: 2 in]
            n525 = local write "Actual B Field (T)"(w1034) -> ()
            n526 = local write "Actual Voltage (V)"(w1033) -> ()
          }
        }
      }
      event "Sweep": Value Change {
        n527 = event-data() -> ("NewVal"=w1062:bool)  [unwired: 1 in, 5 out]
        n528 = case shown="True" w1062 {
          frame False {
          }
          frame True {
            n529 = local read "Measurement File"() -> (w1063:path)
            n530 = Two Button Dialog(message="Do you want to create additional files for the sweeping measurements?" ("string"), 1:"No" ("F button name (\"Cancel\")"), 2:"Yes" ("T button name (\"OK\")")) -> (T button?=w1065:bool)
            n531 = case shown="True" w1065 {
              tunnel: w1063 -> [_ w1070]
              frame False {
                n532 = local write "SaveSweep"(FALSE ("SaveSweep")) -> ()
              }
              frame True {
                n533 = call "Create_sweep_files.vi"("Measurement File"=w1070) -> ("Path 3"=→"Measurement File_dn":path, "Path 2"=→"Measurement File_up":path, "Path"=→"Measurement File_average":path)  [unwired: 8 in]
                "SaveSweep" <- TRUE
              }
            }
          }
        }
      }
      event "Measure Noise": Value Change {
        n534 = event-data() -> ("NewVal"=w1077:bool)  [unwired: 1 in, 5 out]
        n535 = case shown="True" w1077 {
          frame False {
          }
          frame True {
            n536 = local read "Gain (V/A)"() -> (w1082:dbl)
            n537 = call "Noise_measurement.vi"("Gain (V/A)"=w1082, "Cycles"="Cycles", "Lower Cut-Off"="Cut-Off Frequency", "minimum value"="minimum value", "Filter On"="Filter On", "maximum value"="maximum value", "physical channels"="physical channels", "rate"="Rate", "samples per channel"="Samples per channel") -> ("Current (pA) Filtered"=→"Current (pA) Filtered":waveform(dbl), "PSD (pA/Hz^1/2) Peaks Removed"=→"PSD (pA/Hz^1/2) Peaks Removed":cluster{"f0":dbl, "df":dbl, "magnitude":dbl[]}, "Current (pA)"=→"Current (pA)":dbl[], "PSD (pA/Hz^1/2)"=→"PSD (pA/Hz^1/2)":cluster{"f0":dbl, "df":dbl, "magnitude":dbl[]})  [unwired: 3 in]
          }
        }
      }
      event "Calibrate": Value Change {
        n538 = event-data() -> ()  [unwired: 1 in, 6 out]
        n539 = case shown="True" "Calibrate" {
          frame False {
          }
          frame True {
            w1097 = dbl[] []
            n540 = while {
              shift-right: [w1130] -> w1095
              shift-left: dbl[][] [] -> [w1129]
              shift-right: [w1113] -> _
              shift-left: w1097 -> [w1125]
              shift-right: [w1122] -> _
              shift-left: w1097 -> [w1124]
              shift-right: [w1112] -> _
              shift-left: w1097 -> [w1123]
              shift-right: [w1104] -> _
              shift-left: 0.0 ("Set Field out") -> [w1103]
              stop <- w1126 stop-if-true
              n541 = call "Calibtarion.vi"("Dwell Time (ms)"="Dwell Time (ms)", "V array in (V)"=w1125, "I array in (A)"=w1123, "Collected array in"=w1129, "B array in (T)"=w1124, "Set Field (T)"=w1103, "dB"="dB") -> ("Best Linear Fit"=w1114:dbl[], "appended array"=→"appended array":dbl[][], "slope"=→"B/V (T/V)":dbl, "V array out (V)"=w1113:dbl[], "Boolean"=w1128:bool, "I array out (A)"=w1112:dbl[], "intercept 2"=→"I0 (A)":dbl, "Collected array out"=w1130:dbl[][], "intercept"=→"B0 (T)":dbl, "B array Out"=w1122:dbl[], "slope 2"=→"V/I (Ohm)":dbl, "Best Linear Fit 2"=w1119:dbl[], "Set Field out"=w1104:dbl)
              n542 = Bundle("I array out (A)"=w1112, "V array out (V)"=w1113) -> (w1121:T11)  [unwired: 1 in]
              n543 = Bundle("I array out (A)"=w1112, "Best Linear Fit"=w1114) -> (w1115:T12)  [unwired: 1 in]
              n544 = Bundle("V array out (V)"=w1113, "B array Out"=w1122) -> (w1117:T13)  [unwired: 1 in]
              n545 = Bundle("V array out (V)"=w1113, "Best Linear Fit 2"=w1119) -> (w1118:T14)  [unwired: 1 in]
              n546 = Or(x=w1128, y="stop 2") -> (x .or. y?=w1126:bool)
              n547 = Build Array(w1121, w1115) -> (→"V_I":T15)
              n548 = Build Array(w1117, w1118) -> (→"B_V":T16)
            }
            n549 = flat-sequence {
              tunnel: w1095 -> [w1101]
              frame #0 {
                n550 = Two Button Dialog(message="Do you want to save calibration file?") -> (T button?=w1100:bool)  [unwired: 2 in]
                n551 = case shown="True" w1100 {
                  tunnel: w1101 -> [_ w1102]
                  frame False {
                  }
                  frame True {
                    n552 = call-poly <vilib>:"Write Delimited Spreadsheet.vi"("2D data"=w1102) -> ()  [unwired: 13 in, 2 out]
                  }
                }
              }
            }
          }
        }
      }
      event "New Measurement File": Value Change {
        n553 = event-data() -> ()  [unwired: 1 in, 6 out]
        n554 = local read "Sweep"() -> (w1132:bool)
        n555 = Open/Create/Replace File(prompt="Please select measurement file\n", operation (0:open)=T5."replace or create with confirmation") -> (refnum out=w1138:refnum<file>)  [unwired: 4 in, 2 out]
        n556 = local write "refnum out"(w1138) -> ()
        n557 = Refnum to Path(1:w1138) -> (0:w1133:path)
        n558 = case shown="True" w1132 {
          tunnel: w1133 -> [_ w1141]
          frame False {
          }
          frame True {
            n559 = Two Button Dialog(message="Do you want to create additional files for the sweeping measurements?" ("string"), 1:"No" ("F button name (\"Cancel\")"), 2:"Yes" ("T button name (\"OK\")")) -> (T button?=w1143:bool)
            n560 = case shown="False" w1143 {
              tunnel: w1141 -> [_ w1151]
              frame False {
                n561 = local write "SaveSweep"(FALSE ("SaveSweep")) -> ()
              }
              frame True {
                n562 = call "Create_sweep_files.vi"("Measurement File"=w1151) -> ("Path 3"=w1148:path, "Path 2"=w1149:path, "Path"=w1150:path)  [unwired: 8 in]
                n563 = local write "Measurement File_dn"(w1148) -> ()
                n564 = local write "Measurement File_average"(w1150) -> ()
                n565 = local write "Measurement File_up"(w1149) -> ()
                n566 = local write "SaveSweep"(TRUE) -> ()
              }
            }
          }
        }
        n567 = local write "Measurement File"(w1133) -> ()
        n568 = local write "Offset?"(FALSE ("Offset?")) -> ()
        n569 = local write "First?"(TRUE ("First?")) -> ()
      }
      event "Heater On/Off": Value Change {
        n570 = event-data() -> ()  [unwired: 1 in, 6 out]
        n571 = case shown="False" "Heater On/Off" {
          tunnel: w1156 -> [w1161 w1167]
          tunnel: w1155 -> [w1159 w1168]
          tunnel: [w1158 w1166] -> w1154
          frame False {
            n572 = VISA Write(VISA resource name=w1161, write buffer="RANGE,1,0", error in (no error)=w1159) -> (error out=w1158:errorcluster)  [unwired: 2 out]
          }
          frame True {
            n573 = Number To Decimal String(number="Heater Range") -> (decimal integer string=w1164:string)  [unwired: 1 in]
            n574 = Concatenate Strings("RANGE,1," ("write buffer"), w1164) -> (w1162:string)
            n575 = VISA Write(VISA resource name=w1167, write buffer=w1162, error in (no error)=w1168) -> (error out=w1166:errorcluster)  [unwired: 2 out]
          }
        }
      }
      event "Set temperature (K)": Value Change {
        n576 = event-data() -> ()  [unwired: 1 in, 6 out]
        n577 = local read "Set temperature (K)"() -> (w1174:dbl)
        n578 = Number To Fractional String(number=w1174, precision (6)=i16 3) -> (F-format string=w1177:string)  [unwired: 2 in]
        n579 = Concatenate Strings("SETP 1," ("write buffer"), w1177) -> (w1175:string)
        n580 = VISA Write(VISA resource name=w1171, write buffer=w1175, error in (no error)=w1173) -> (error out=w1172:errorcluster)  [unwired: 2 out]
      }
      event "Temp Ramping Rate (K/min)": Value Change {
        n581 = event-data() -> ()  [unwired: 1 in, 6 out]
        n582 = local read "Temp Ramping Rate (K/min)"() -> (w1181:dbl)
        n583 = Number To Fractional String(number=w1181, precision (6)=i16 1) -> (F-format string=w1187:string)  [unwired: 2 in]
        n584 = Concatenate Strings("RAMP 1,1," ("string"), w1187) -> (w1186:string)
        n585 = VISA Write(VISA resource name=w1184, write buffer=w1186, error in (no error)=w1183) -> (error out=w1182:errorcluster)  [unwired: 2 out]
      }
      event "Heater Range": Value Change {
        n586 = event-data() -> ()  [unwired: 1 in, 6 out]
        n587 = local read "Heater On/Off"() -> (w1193:bool)
        n588 = case shown="True" w1193 {
          tunnel: w1192 -> [w1194 w1199]
          tunnel: [w1194 w1198] -> w1191
          tunnel: w1189 -> [_ w1197]
          frame False {
          }
          frame True {
            n589 = local read "Heater Range"() -> (w1195:enum16{"Off", "Low", "Medium", "High"})
            n590 = Number To Decimal String(number=w1195) -> (decimal integer string=w1201:string)  [unwired: 1 in]
            n591 = Concatenate Strings("RANGE,1," ("write buffer"), w1201) -> (w1200:string)
            n592 = VISA Write(VISA resource name=w1197, write buffer=w1200, error in (no error)=w1199) -> (error out=w1198:errorcluster)  [unwired: 2 out]
          }
        }
      }
    }
    n593 = Reciprocal(x="Sampling rate (Hz)") -> (1/x=w869:dbl)
    n594 = Multiply(x=w869, y=1000.0) -> (x*y=w867:dbl)
    n595 = Wait Until Next ms Multiple(millisecond multiple=w867) -> ()  [unwired: 1 out]
  }
  n596 = local read "Max Field (T)"() -> (w57:dbl)
  n597 = local read "Min Field (T)"() -> (w59:dbl)
  n598 = local read "dB (T)"() -> (w58:dbl)
  n599 = Divide(x=w57, y=w58) -> (x/y=w60:dbl)
  n600 = for {
    N: w60 -> [_]
    tunnel: w58 -> [w1206]
    tunnel: [w1203] -> w20 mode=indexing
    tunnel: w59 -> [w1204]
    tunnel: [0.0] -> _ mode=indexing
    i -> [w1207]
    n601 = Multiply(x=w1207, y=w1206) -> (x*y=w1205:dbl)
    n602 = Add(x=w1205, y=w1204) -> (x+y=w1203:dbl)
  }
  n603 = Multiply(x=w20, y=0.0) -> (x*y=w17:dbl[])
  n604 = Array Size(array=w17) -> (size(s)=w16:i32)
  n605 = Decrement(x=w16) -> (x-1=w15:i32)
  n606 = local write "B array"(w20) -> ()
  n607 = Array Subset(array=w17, length=w15) -> (w14:dbl[])  [unwired: 1 in]
  n608 = Build Array(w17, w17) -> (w18:dbl[][])
  n609 = local write "Averaged I(B)"(w18) -> ()
  n610 = Build Array(w14, w14) -> (w13:dbl[][])
  n611 = local write "Averaged P(B)"(w13) -> ()
  n612 = local write "Averaged dt"(w13) -> ()
  n613 = local read "Lake Shore"() -> (w70:refnum<visa-resource-name>)
  n614 = local read "IV converter"() -> (w86:refnum<visa-resource-name>)
  n615 = local read "Magnetic Field"() -> (w85:refnum<visa-resource-name>)
  n616 = VISA Close(VISA resource name=w86, error in (no error)=w88) -> (error out=w89:errorcluster)
  n617 = VISA Close(VISA resource name=w85, error in (no error)=w89) -> (error out=w87:errorcluster)
  n618 = Release Queue(queue=w95, error in (no error)=w87) -> (error out=w83:errorcluster)  [unwired: 1 in, 2 out]
  n619 = Merge Errors(w83, w82) -> (w84:errorcluster)
  n620 = VISA Close(VISA resource name=w70, error in (no error)=w84) -> (error out=w81:errorcluster)
  n621 = local read "refnum out"() -> (w79:refnum<file>)
  n622 = Close File(refnum=w79, error in=w81) -> (error out=w80:errorcluster)  [unwired: 1 out]
  n623 = call <vilib>:"Simple Error Handler.vi"("error in (no error)"=w80) -> ()  [unwired: 4 in, 5 out]
  "i" <- w50
  "j" <- w50
